vi "单板信息.vi"(11 "VIC_Receive":refnum<vi>) -> ()   [LabVIEW 2013]
panel:
  in  "从板板号 2":u8=1 caption="从板板号" min=1 max=30
  out "滑动杆":dbl(slide)=90.0 caption="SOC" scale=0.0..100.0 scale format="%#_6f"
  out "5":T1
  out "4":T2
  out "3":T3
  out "2":T4
  out "平均电流(A)":dbl
  out "外总压(V)":dbl
  out "总电流(A)":dbl
  out "协议是否公开":string="是"
  out "波特率":string="500Kbps"
  out "应用类型":string
  out "协议版本号":string
  out "SOH":dbl(slide)=30.0 scale=0.0..100.0 scale format="%#_6f"
  in  "刷新":bool
  in  "布尔 3":bool
  out "故障信息":string
  out "最小内阻位置":i32
  out "最大内阻位置":i32
  out "最小内阻":dbl
  out "最大内阻":dbl
  out "最低温度位置":i32
  out "最高温度位置":i32
  out "最低温度":dbl
  out "最高温度":dbl
  out "最低电压位置":i32
  out "最高电压位置":i32
  out "最低电压":dbl
  out "最高电压":dbl
  in  "主界面选项":enum32{"单选选项1", "单选选项2", "单选选项2 2"}(radio)
  in  "继电器状态 2":string[][](table)=[["RL1_ST", "", "RL5_ST"], ["RL2_ST", "", "RL6_ST"], ["RL3_ST", "", "RL7_ST"], ["RL4_ST", "", "RL8_ST"]]
  out "快换帧":T5
  out "从板参数":T6={"总电压"=0.0, "总电流"=0.0, "外总压"=0.0, "平均电流"=0.0, "SOC"=60.0, "SOH"=60.0, "最高电压"=0.0, "位置"=0.0, "最低电压"=0.0, "位置"=0.0, "压差"=0.0, "最高温度"=0.0, "位置"=0.0, "最低温度"=0.0, "位置"=0.0, "最大内阻"=0.0, "位置"=0.0, "最小内阻"=0.0, "位置"=0.0, "故障信息"="", "协议版本号"="", "应用类型"="", "波特率"="", "协议是否公开"="", "电池运行状态"="", "电池充满标志位"="", "Life:"=25.0} {"SOH" scale=0.0..100.0 scale format="%#.0f"; "SOC" scale=0.0..100.0 scale format="%#.0f"}
  out "Life:":dbl=25.0
  out "状态":bool
  out "高压板参数":T7={"总电压"=0.0, "总电流"=0.0, "外总压"=0.0, "平均电流"=0.0, "功率"=0.0, "总充电安时"=0.0, "总放电安时"=0.0, "故障信息"="", "协议版本号"="", "应用类型"="", "波特率"="", "协议是否公开"="", "电池运行状态"="", "Life:"=25.0, "正绝缘电阻"=0.0, "负绝缘电阻"=0.0} {"负绝缘电阻" format="%#.0f"; "正绝缘电阻" format="%#.0f"; "总放电安时" format="%#.0f"; "总充电安时" format="%#.0f"}
  out "继电器颜色":u32[](array[colorbox])
  out "继电器状态":string[](array[string])
  in  "选项卡控件":enum32{"从板监控", "从板信息2", "电压温度", "高压板监控"}(tab)=enum."从板信息2"
  out "从板参数":T8={"最高电压"=0.0, "位置1"=0.0, "最低电压"=0.0, "位置2"=0.0, "压差"=0.0, "最高温度"=0.0, "位置3"=0.0, "最低温度"=0.0, "位置4"=0.0, "温差"=0.0, "最高内阻"=0.0, "位置5"=0.0, "最低内阻"=0.0, "位置6"=0.0, "故障信息"="00", "最大充电总电压"=0.0, "最大充电电流"=0.0, "充电总安时"=0.0, "SOH 2"=0.0, "RL1_ST(fan)"="", "RL2_ST(heat)"="", "RL3_ST"="", "RL4_ST"="", "RL5_ST"="", "RL6_ST"="", "RL7_ST"="", "RL8_ST"=""}
  out "电池充满标志位":string="是"
  out "电池运行状态":string="00"
  out "总电压(V)":dbl
  out "硬件故障":string[][](array[string])
  in  "欠压":u16(ring)
  in  "过压":u16(ring)
  in  "无效":u16(ring)
  in  "故障":u16(ring)
  in  "正常":u16(ring)
  out "供电电源电压(V)":string="0"
  out "内网总线负载率":string="0"
  out "供电电源状态":u16(ring)=1
  out "Flash存储器状态":u16(ring)
  out "外部EE存储器状态":u16(ring)=1
  out "内部EE存储器状态":u16(ring)=3
  out "系统时钟状态":u16(ring)
  out "内部总电压检测模块状态":u16(ring)
  out "外部总电压检测模块状态":u16(ring)
  out "绝缘检测模块状态":u16(ring)
  out "电流模块模块状态":u16(ring)=1 caption="电流检测模块状态"
  out "电池充电均衡模块状态":u16(ring)
  out "电池放电均衡模块状态":u16(ring)=1
  out "温度模块检测状态":u16(ring)=3 caption="温度检测模块状态"
  out "电压模块检测状态":u16(ring) caption="电压检测模块状态"
  in  "偏差":dbl=10.0 format="%#.0f"
  in  "温度基准":dbl=25.0 format="%#.0f"
  in  "布尔 2":bool caption="判定"
  in  "偏差":dbl=0.05 format="%.3f"
  in  "电压基准":dbl=3.7 format="%.3f"
  in  "布尔":bool caption="判定"
  out "1":T9 {"第12串" format="%#.2f"; "第11串" format="%#.2f"; "第10串" format="%#.2f"; "第9串" format="%#.2f"; "第8串" format="%#.2f"; "第7串" format="%#.2f"; "第6串" format="%#.2f"; "第5串" format="%#.2f"; "第4串" format="%#.2f"; "第3串" format="%#.2f"; "第2串" format="%#.2f"; "第1串" format="%#.2f"}
  out "1 7":T1 {"第60串" format="%.3f"; "第59串" format="%.3f"; "第58串" format="%.3f"; "第57串" format="%.3f"; "第56串" format="%.3f"; "第55串" format="%.3f"; "第54串" format="%.3f"; "第53串" format="%.3f"; "第52串" format="%.3f"; "第51串" format="%.3f"; "第50串" format="%.3f"; "第49串" format="%.3f"}
  out "1 6":T2 {"第48串" format="%.3f"; "第47串" format="%.3f"; "第46串" format="%.3f"; "第45串" format="%.3f"; "第44串" format="%.3f"; "第43串" format="%.3f"; "第42串" format="%.3f"; "第41串" format="%.3f"; "第40串" format="%.3f"; "第39串" format="%.3f"; "第38串" format="%.3f"; "第37串" format="%.3f"}
  out "1 4":T3 {"第36串" format="%.3f"; "第35串" format="%.3f"; "第34串" format="%.3f"; "第33串" format="%.3f"; "第32串" format="%.3f"; "第31串" format="%.3f"; "第30串" format="%.3f"; "第29串" format="%.3f"; "第28串" format="%.3f"; "第27串" format="%.3f"; "第26串" format="%.3f"; "第25串" format="%.3f"}
  out "1 3":T4 {"第24串" format="%.3f"; "第23串" format="%.3f"; "第22串" format="%.3f"; "第21串" format="%.3f"; "第20串" format="%.3f"; "第19串" format="%.3f"; "第18串" format="%.3f"; "第17串" format="%.3f"; "第16串" format="%.3f"; "第15串" format="%.3f"; "第14串" format="%.3f"; "第13串" format="%.3f"}
  out "1 102":T9 {"第12串" format="%.3f"; "第11串" format="%.3f"; "第10串" format="%.3f"; "第9串" format="%.3f"; "第8串" format="%.3f"; "第7串" format="%.3f"; "第6串" format="%.3f"; "第5串" format="%.3f"; "第4串" format="%.3f"; "第3串" format="%.3f"; "第2串" format="%.3f"; "第1串" format="%.3f"}
  out "高压板监控":T10={"总电压"=0.0, "总电流"=0.0, "外总压"=0.0, "平均电流"=0.0, "功率"=0.0, "总充电安时"=0.0, "总放电安时"=0.0, "正绝缘电阻"=0.0, "负绝缘电阻"=0.0, "版本协议号"="V1.2.34", "应用类型"="纯电动", "波特率"="500Kbps", "协议是否公开"="是", "故障信息"="00", "电池运行情况"="00"}
  in  "VCI_Receive":T11 {"Rsv3" max=0 format="%x"; "Rsv2" min=101 format="%x"; "Rsv1" format="%x"; "Data8" format="%x"; "Data7" format="%x"; "Data6" format="%x"; "Data5" format="%x"; "Data4" format="%x"; "Data3" format="%x"; "Data2" format="%x"; "Data1" format="%x"; "DataLen" format="%x"; "ExternFlag" format="%x"; "RemoteFlag" format="%x"; "SendType" format="%x"; "TimeFlag" format="%x"; "TimeStamp" format="%x"; "ID" format="%x"}
  in  "停止":bool
  out "单选选项2":bool
  # "从板继电器"
  # "Change frame"
  # "图例"
  # "CellV"
  # "Temp"
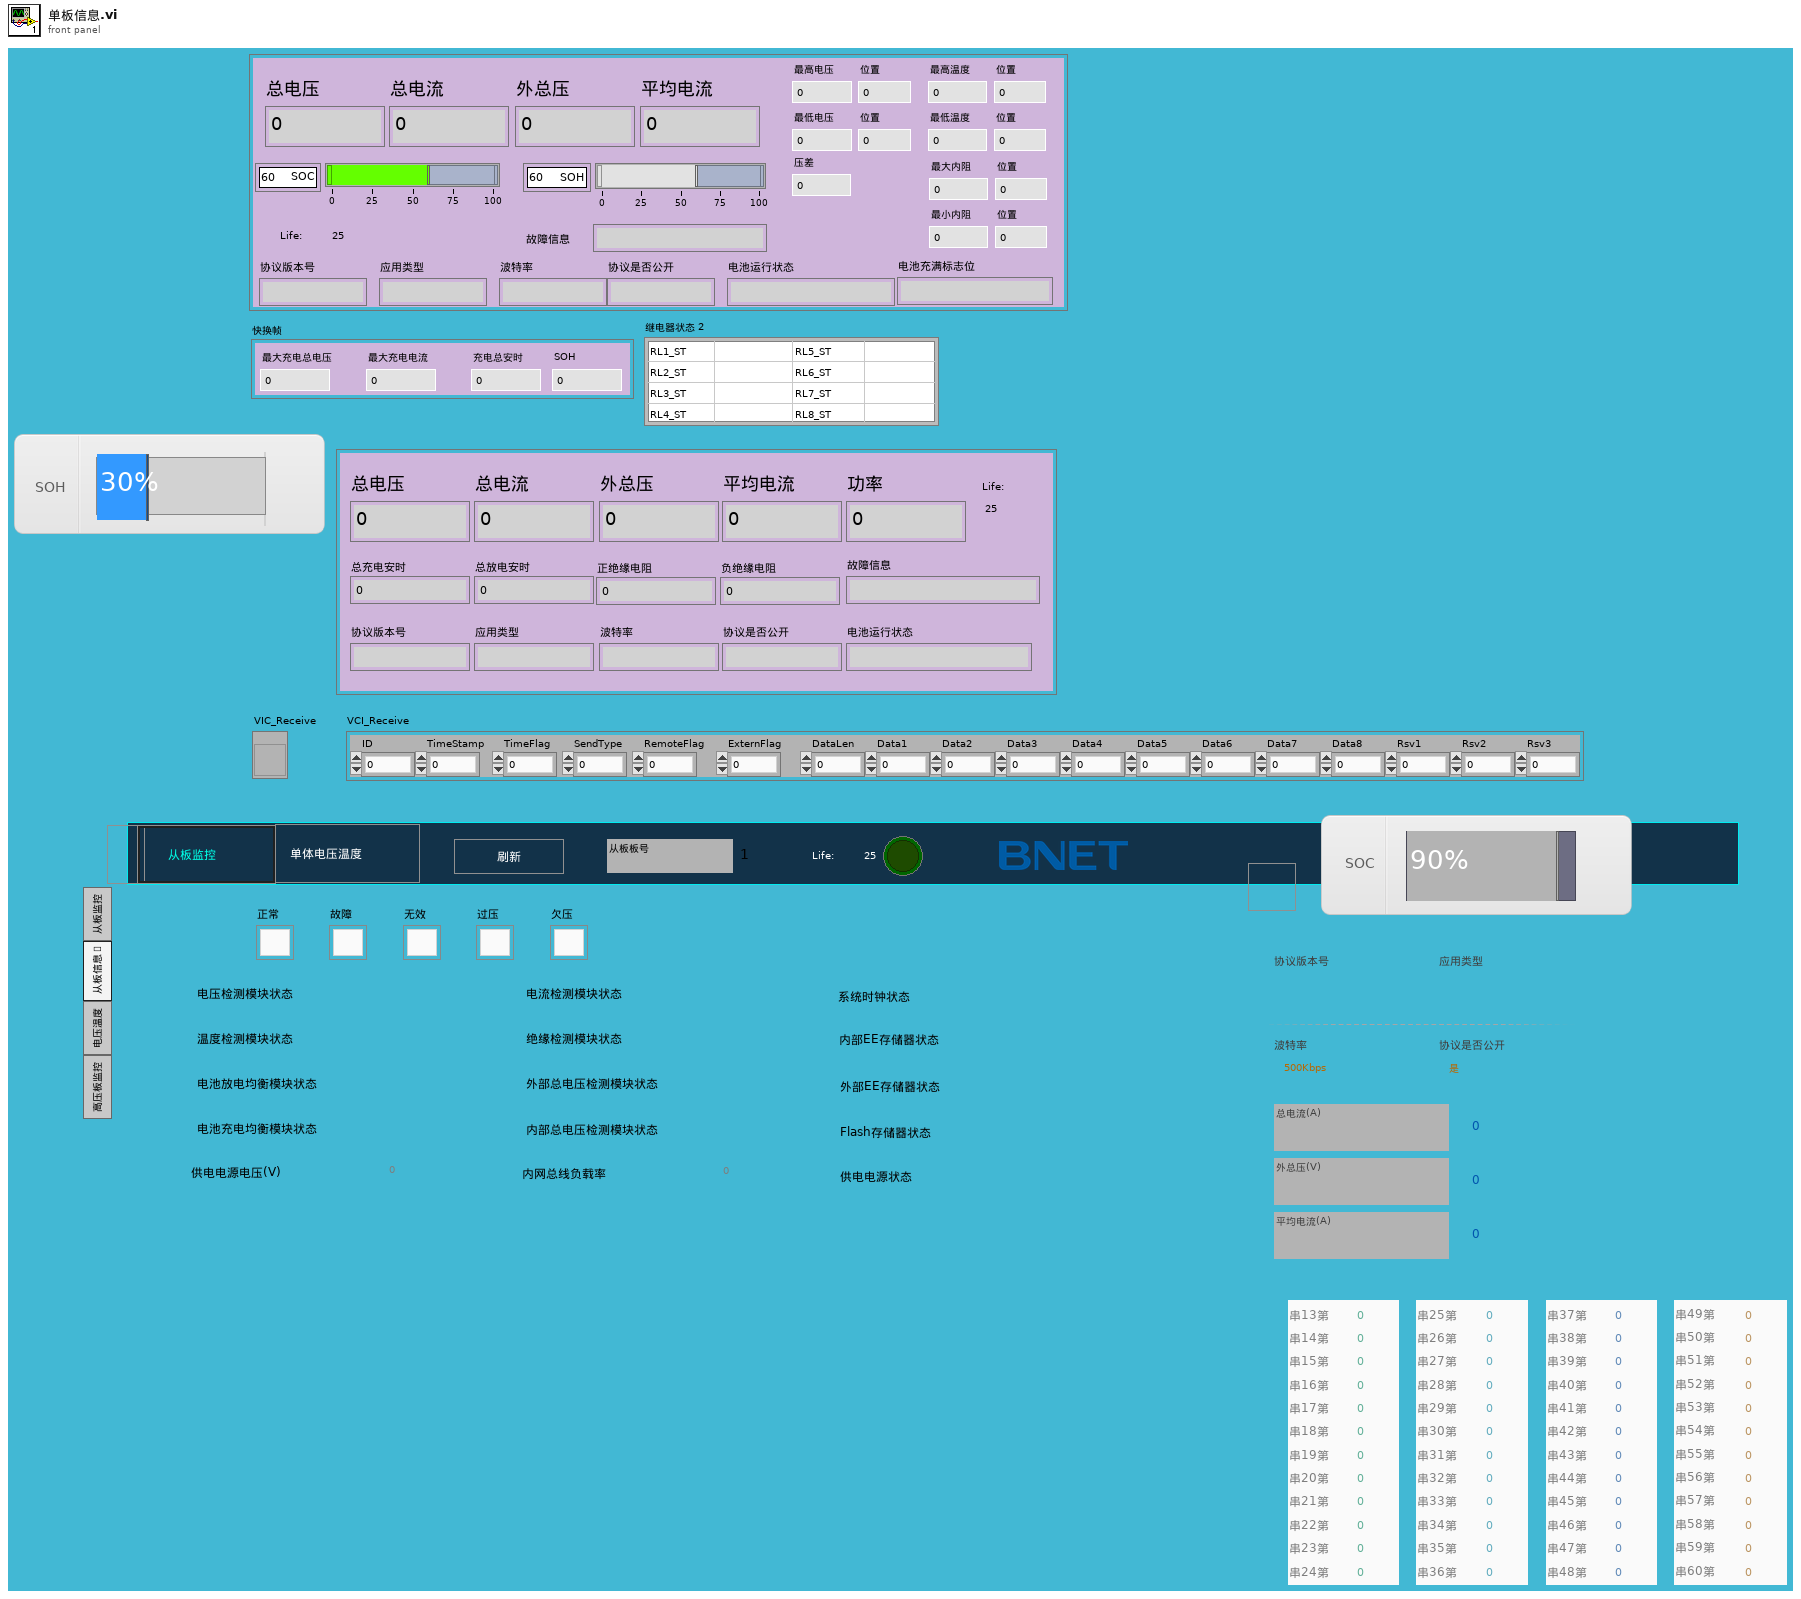
[diagram p1: front panel]
types:
  T1 = cluster{"第49串":dbl, "第50串":dbl, "第51串":dbl, "第52串":dbl, "第53串":dbl, "第54串":dbl, "第55串":dbl, "第56串":dbl, "第57串":dbl, "第58串":dbl, "第59串":dbl, "第60串":dbl}
  T2 = cluster{"第37串":dbl, "第38串":dbl, "第39串":dbl, "第40串":dbl, "第41串":dbl, "第42串":dbl, "第43串":dbl, "第44串":dbl, "第45串":dbl, "第46串":dbl, "第47串":dbl, "第48串":dbl}
  T3 = cluster{"第25串":dbl, "第26串":dbl, "第27串":dbl, "第28串":dbl, "第29串":dbl, "第30串":dbl, "第31串":dbl, "第32串":dbl, "第33串":dbl, "第34串":dbl, "第35串":dbl, "第36串":dbl}
  T4 = cluster{"第13串":dbl, "第14串":dbl, "第15串":dbl, "第16串":dbl, "第17串":dbl, "第18串":dbl, "第19串":dbl, "第20串":dbl, "第21串":dbl, "第22串":dbl, "第23串":dbl, "第24串":dbl}
  T5 = cluster{"SOH":dbl, "充电总安时":dbl, "最大充电电流":dbl, "最大充电总电压":dbl}
  T6 = cluster{"总电压":dbl, "总电流":dbl, "外总压":dbl, "平均电流":dbl, "SOC":dbl, "SOH":dbl, "最高电压":dbl, "位置":dbl, "最低电压":dbl, "位置":dbl, "压差":dbl, "最高温度":dbl, "位置":dbl, "最低温度":dbl, "位置":dbl, "最大内阻":dbl, "位置":dbl, "最小内阻":dbl, "位置":dbl, "故障信息":string, "协议版本号":string, "应用类型":string, "波特率":string, "协议是否公开":string, "电池运行状态":string, "电池充满标志位":string, "Life:":dbl}
  T7 = cluster{"总电压":dbl, "总电流":dbl, "外总压":dbl, "平均电流":dbl, "功率":dbl, "总充电安时":dbl, "总放电安时":dbl, "故障信息":string, "协议版本号":string, "应用类型":string, "波特率":string, "协议是否公开":string, "电池运行状态":string, "Life:":dbl, "正绝缘电阻":dbl, "负绝缘电阻":dbl}
  T8 = cluster{"最高电压":dbl, "位置1":dbl, "最低电压":dbl, "位置2":dbl, "压差":dbl, "最高温度":dbl, "位置3":dbl, "最低温度":dbl, "位置4":dbl, "温差":dbl, "最高内阻":dbl, "位置5":dbl, "最低内阻":dbl, "位置6":dbl, "故障信息":string, "最大充电总电压":dbl, "最大充电电流":dbl, "充电总安时":dbl, "SOH 2":dbl, "RL1_ST(fan)":string, "RL2_ST(heat)":string, "RL3_ST":string, "RL4_ST":string, "RL5_ST":string, "RL6_ST":string, "RL7_ST":string, "RL8_ST":string}
  T9 = cluster{"第1串":dbl, "第2串":dbl, "第3串":dbl, "第4串":dbl, "第5串":dbl, "第6串":dbl, "第7串":dbl, "第8串":dbl, "第9串":dbl, "第10串":dbl, "第11串":dbl, "第12串":dbl}
  T10 = cluster{"总电压":dbl, "总电流":dbl, "外总压":dbl, "平均电流":dbl, "功率":dbl, "总充电安时":dbl, "总放电安时":dbl, "正绝缘电阻":dbl, "负绝缘电阻":dbl, "版本协议号":string, "应用类型":string, "波特率":string, "协议是否公开":string, "故障信息":string, "电池运行情况":string}
  T11 = cluster{"ID":u32, "TimeStamp":u32, "TimeFlag":u8, "SendType":u8, "RemoteFlag":u8, "ExternFlag":u8, "DataLen":u8, "Data1":u8, "Data2":u8, "Data3":u8, "Data4":u8, "Data5":u8, "Data6":u8, "Data7":u8, "Data8":u8, "Rsv1":u8, "Rsv2":u8, "Rsv3":u8}
  T12 = cluster{dbl, dbl, dbl, dbl, dbl, dbl, dbl, dbl, dbl, dbl, dbl, dbl, dbl, dbl, "故障信息":string, dbl, dbl, dbl, dbl, "RL1_ST":string, "RL2_ST":string, "RL3_ST":string, "RL4_ST":string, "RL5_ST":string, "RL6_ST":string, "RL7_ST":string, "RL8_ST":string}
  T13 = enum32{"Invalid", "Standard", "Closed", "Hidden", "Minimized", "Maximized"}
  T14 = cluster{"[0]":dbl, "[1]":dbl, "[2]":dbl, "[3]":dbl, "[4]":dbl, "[5]":dbl, "[6]":dbl, "[7]":dbl, "[8]":dbl, "[9]":dbl, "[10]":dbl, "[11]":dbl}
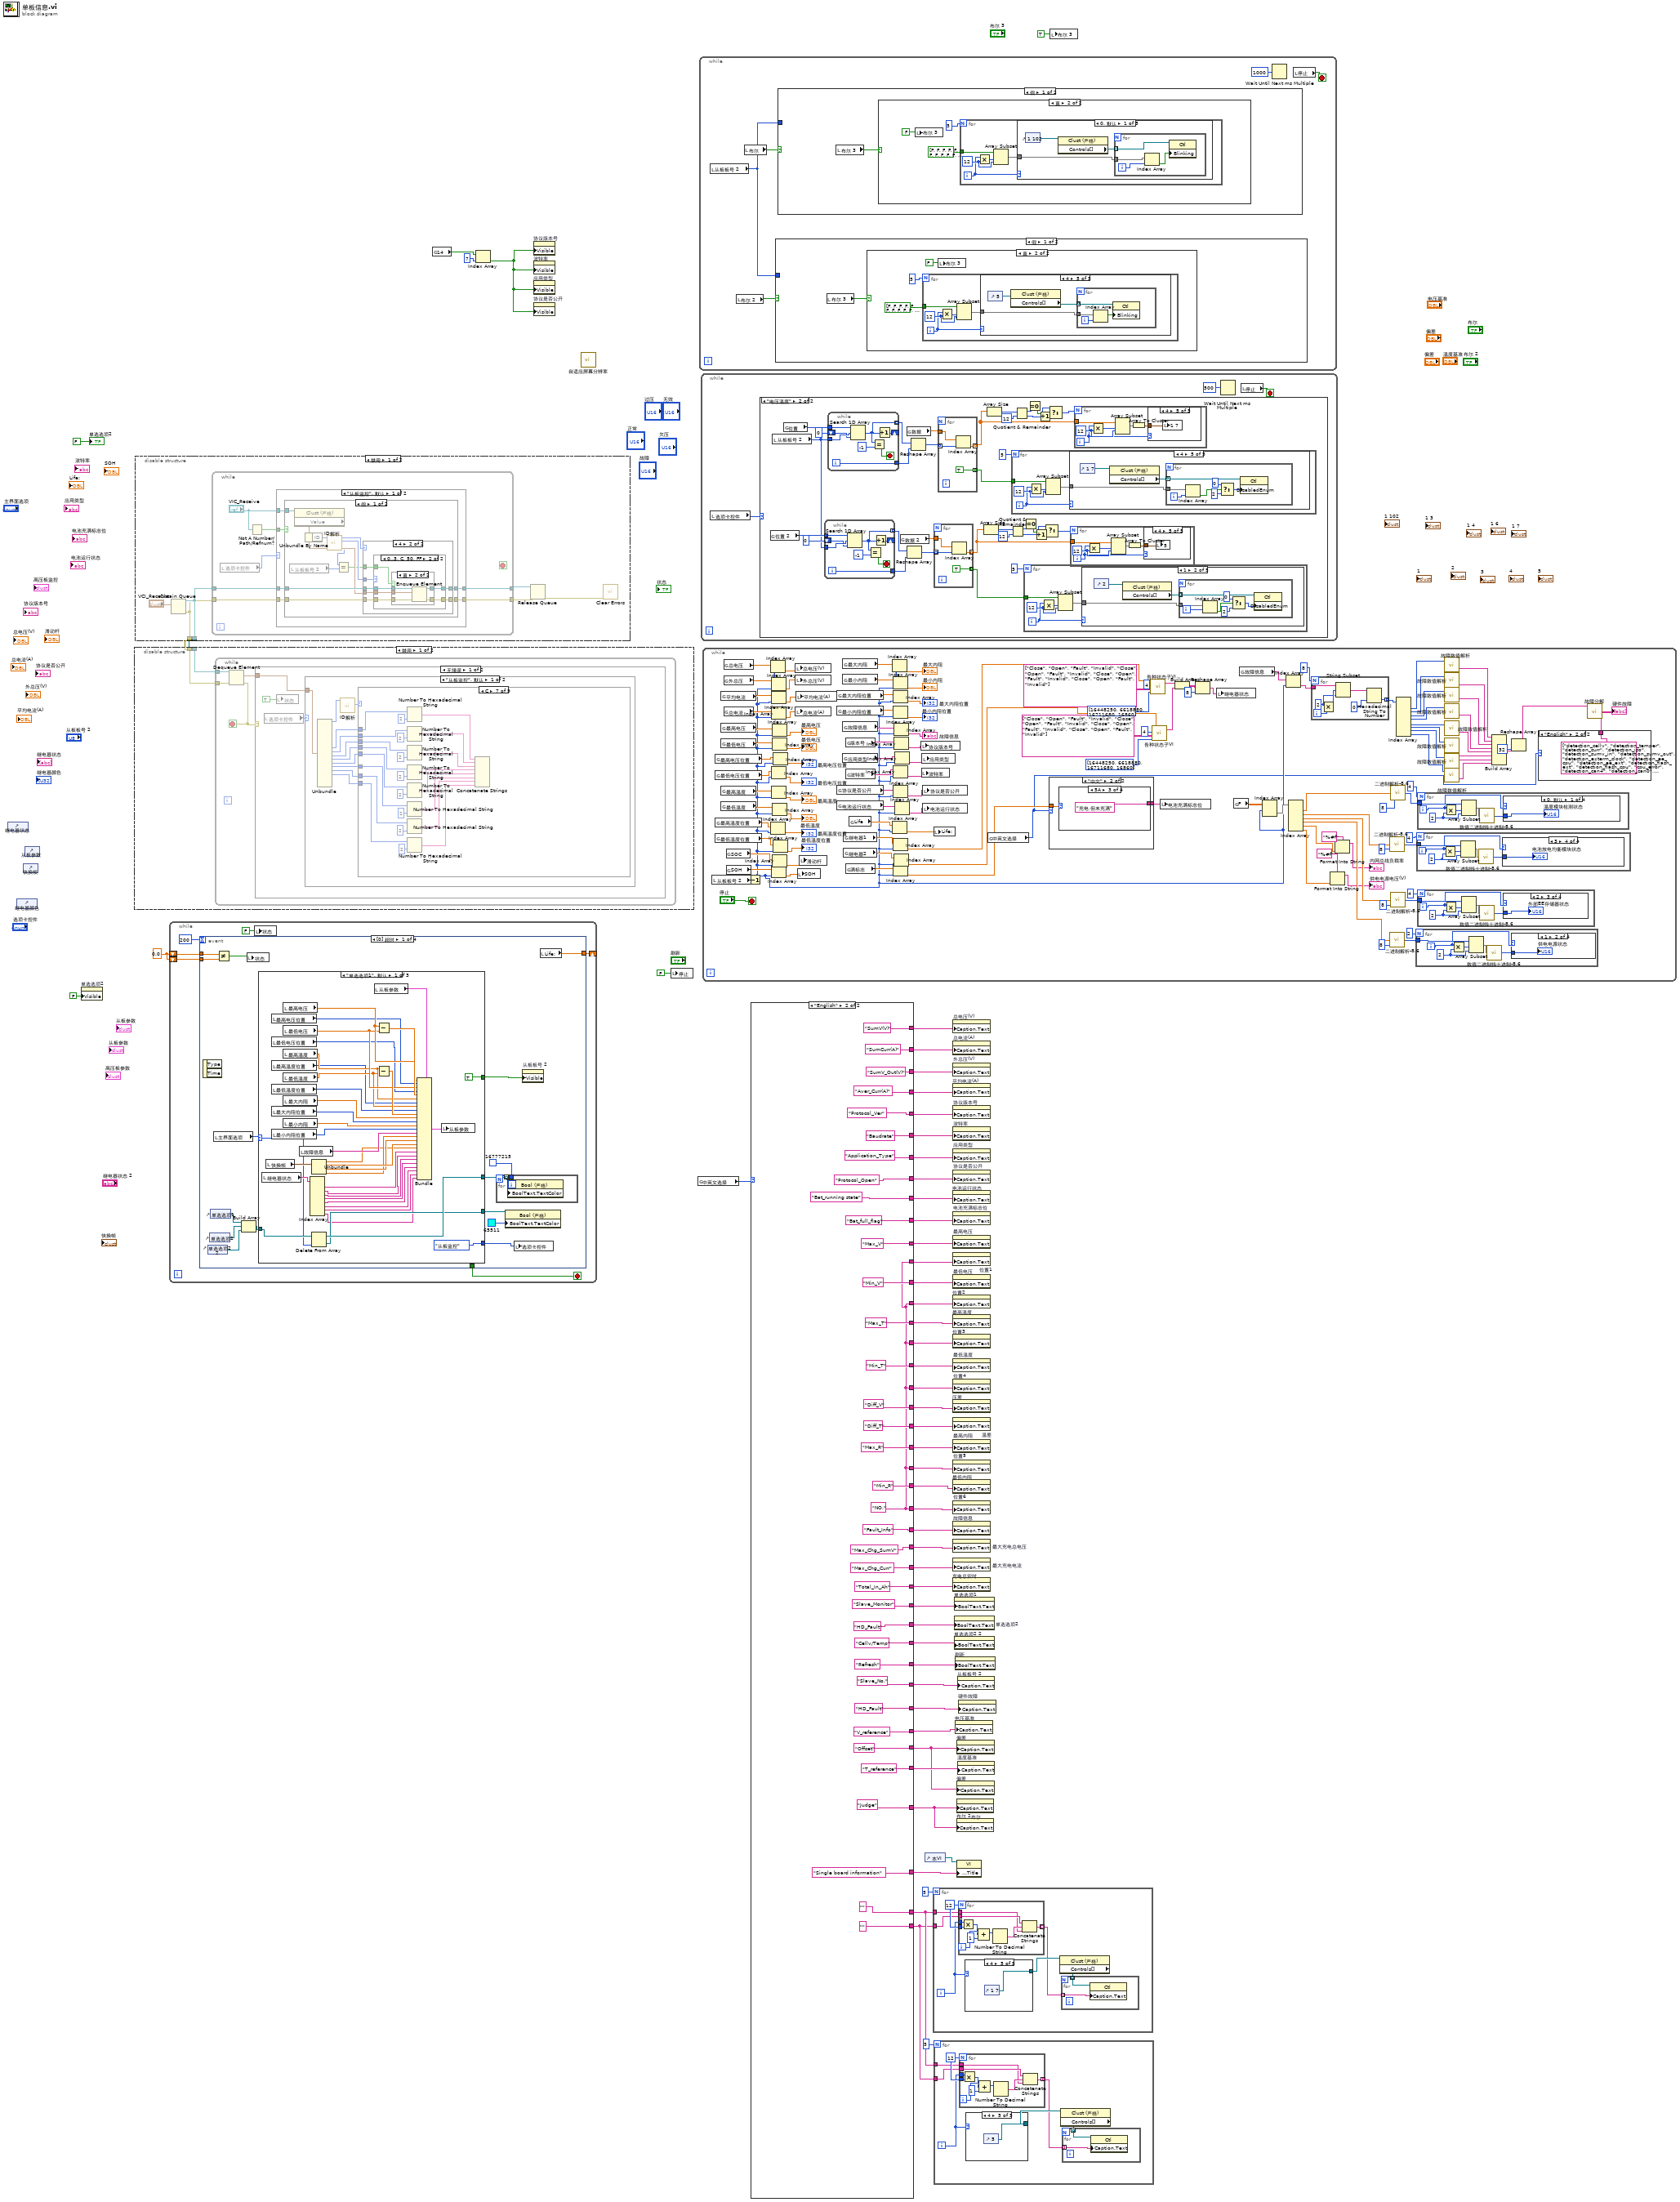
[diagram p0: block diagram]
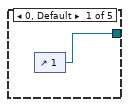
[diagram p2: hidden frame]
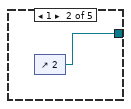
[diagram p3: hidden frame]
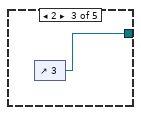
[diagram p4: hidden frame]
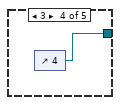
[diagram p5: hidden frame]
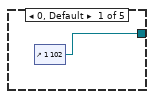
[diagram p6: hidden frame]
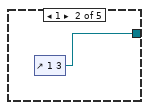
[diagram p7: hidden frame]
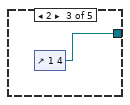
[diagram p8: hidden frame]
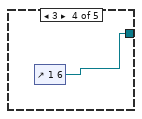
[diagram p9: hidden frame]
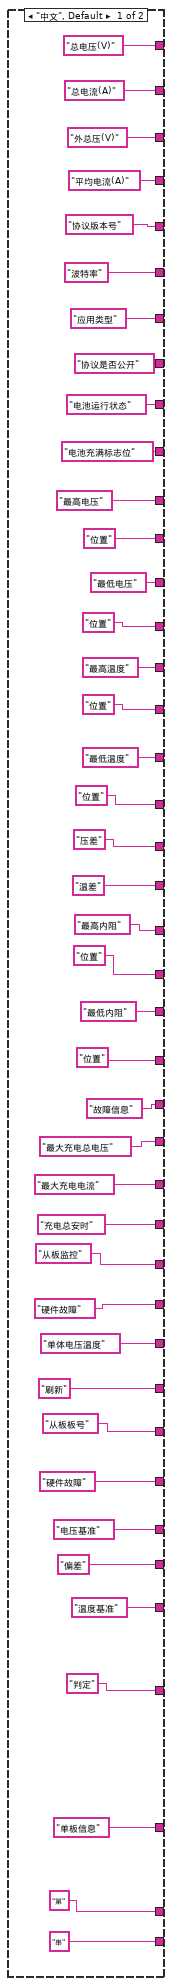
[diagram p10: hidden frame]
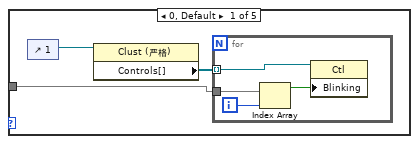
[diagram p12: hidden frame]
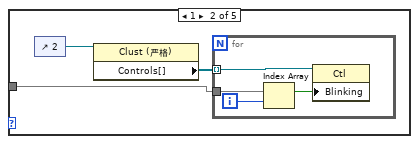
[diagram p13: hidden frame]
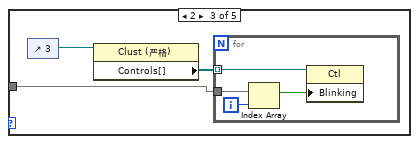
[diagram p14: hidden frame]
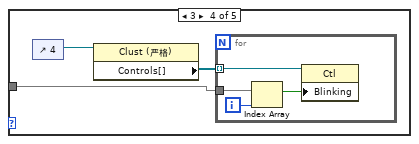
[diagram p15: hidden frame]
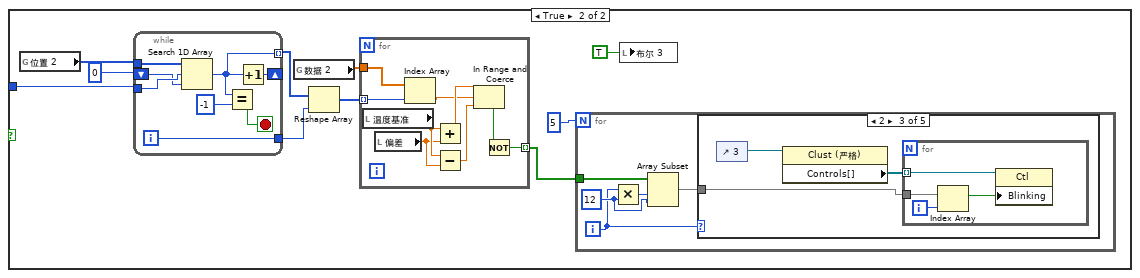
[diagram p16: hidden frame]
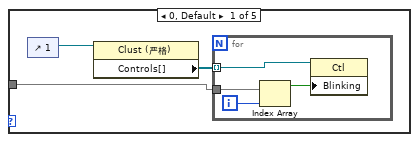
[diagram p17: hidden frame]
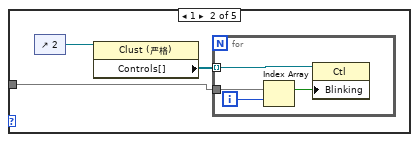
[diagram p18: hidden frame]
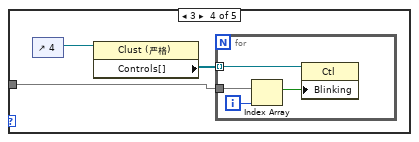
[diagram p19: hidden frame]
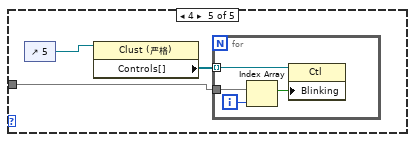
[diagram p20: hidden frame]
diagram:
  w50 = 0.0 ("Life:")
  n1 = control-ref of="继电器状态"() -> ()  [unwired: 1 out]
  n2 = control-ref of="继电器颜色"() -> ()  [unwired: 1 out]
  n3 = control-ref of="快换帧"() -> ()  [unwired: 1 out]
  n4 = control-ref of="从板参数"() -> ()  [unwired: 1 out]
  n5 = property on="单选选项2" class="Bool (严格)"("Visible"=FALSE ("可见")) -> ()  [unwired: 2 in, 2 out]
  n6 = disable-structure shown="禁用" {
    disable-tunnel: [w60 _] -> w55
    disable-tunnel: [w59 _] -> w54
    frame Disabled {
      n7 = Obtain Queue(element data type="VCI_Receive") -> (queue out=w60:refnum<queue>, error out=w59:errorcluster)  [unwired: 4 in, 1 out]
      n8 = while {
        tunnel: w60 -> [w67]
        tunnel: w59 -> [w66]
        tunnel: [w65] -> w58
        tunnel: [w64] -> w57
        stop <- w68 stop-if-true
        n9 = local read "选项卡控件"() -> (w62:enum32{"从板监控", "从板信息2", "电压温度", "高压板监控"})
        n10 = Not A Number/Path/Refnum?(number/path/refnum="VIC_Receive") -> (NaN/Path/Refnum?=w63:bool)
        n11 = case shown="\"从板监控\", 默认" w62 {
          tunnel: "VIC_Receive" -> [w75 w120]
          tunnel: w67 -> [w74 w119]
          tunnel: w66 -> [w73 w118]
          tunnel: [w72 w117] -> w65
          tunnel: [w71 w116] -> w64
          tunnel: w63 -> [w70 w115]
          frame "从板监控", Default {
            n12 = case shown="假" w70 {
              tunnel: w74 -> [w86 w114]
              tunnel: w73 -> [w85 w113]
              tunnel: [w83 w114] -> w72
              tunnel: [w82 w113] -> w71
              tunnel: w75 -> [w81 _]
              frame False {
                n13 = local read "从板板号 2"() -> (w76:u8)
                n14 = property class="Clust (严格)"(reference=w81) -> ("Value"=w84:T11)  [unwired: 1 in, 2 out]
                n15 = Unbundle By Name(w84) -> ("ID"=w87:u32)
                n16 = call "ID解析.vi"("ID"=w87) -> ("SA(4)"=w78:i32, "PF(2)"=w79:i32, "PDU(1)"=w80:i32)  [unwired: 8 out]
                n17 = Equal?(x=w78, y=w76) -> (x = y?=w77:bool)
                n18 = case shown="4" w80 {
                  tunnel: w86 -> [w89 w96]
                  tunnel: w85 -> [w88 w95]
                  tunnel: w84 -> [_ w94]
                  tunnel: [w89 w93] -> w83
                  tunnel: [w88 w92] -> w82
                  tunnel: w79 -> [_ w91]
                  tunnel: w77 -> [_ w90]
                  frame 0, Default {
                  }
                  frame 4 {
                    n19 = case shown="0..3, C, 50, FF" w91 {
                      tunnel: w96 -> [w98 w104]
                      tunnel: w95 -> [w97 w103]
                      tunnel: w94 -> [_ w102]
                      tunnel: [w98 w101] -> w93
                      tunnel: [w97 w100] -> w92
                      tunnel: w90 -> [_ w99]
                      frame 153, Default {
                      }
                      frame 0..3, 12, 80, 255 {
                        n20 = case shown="真" w99 {
                          tunnel: w104 -> [w106 w111]
                          tunnel: w103 -> [w105 w110]
                          tunnel: w102 -> [_ w109]
                          tunnel: [w106 w108] -> w101
                          tunnel: [w105 w107] -> w100
                          frame False {
                          }
                          frame True {
                            n21 = Enqueue Element(queue=w111, element=w109, error in (no error)=w110) -> (queue out=w108:refnum<queue>, error out=w107:errorcluster)  [unwired: 2 out]
                          }
                        }
                      }
                    }
                  }
                }
              }
              frame True {
                n22 = Wait Until Next ms Multiple(millisecond multiple=u32 100 ("毫秒倍数")) -> ()  [unwired: 1 out]
              }
            }
          }
          frame "高压板监控" {
            n23 = case shown="假" w115 {
              tunnel: w119 -> [w132 w160]
              tunnel: w118 -> [w131 w159]
              tunnel: [w129 w160] -> w117
              tunnel: [w128 w159] -> w116
              tunnel: w120 -> [w127 _]
              frame False {
                n24 = property class="Clust (严格)"(reference=w127) -> ("Value"=w130:T11)  [unwired: 1 in, 2 out]
                n25 = Unbundle By Name(w130) -> ("ID"=w133:u32)
                n26 = call "ID解析.vi"("ID"=w133) -> ("SA(4)"=w124:i32, "PF(2)"=w125:i32, "PDU(1)"=w126:i32)  [unwired: 8 out]
                n27 = Equal?(x=w124, y=62) -> (x = y?=w123:bool)
                n28 = case shown="4" w126 {
                  tunnel: w132 -> [w135 w142]
                  tunnel: w131 -> [w134 w141]
                  tunnel: w130 -> [_ w140]
                  tunnel: [w135 w139] -> w129
                  tunnel: [w134 w138] -> w128
                  tunnel: w125 -> [_ w137]
                  tunnel: w123 -> [_ w136]
                  frame 0, Default {
                  }
                  frame 4 {
                    n29 = case shown="0, 5, 8, C, FF" w137 {
                      tunnel: w142 -> [w144 w150]
                      tunnel: w141 -> [w143 w149]
                      tunnel: w140 -> [_ w148]
                      tunnel: [w144 w147] -> w139
                      tunnel: [w143 w146] -> w138
                      tunnel: w136 -> [_ w145]
                      frame 153, Default {
                      }
                      frame 0, 5, 8, 12, 255 {
                        n30 = case shown="真" w145 {
                          tunnel: w150 -> [w152 w157]
                          tunnel: w149 -> [w151 w156]
                          tunnel: w148 -> [_ w155]
                          tunnel: [w152 w154] -> w147
                          tunnel: [w151 w153] -> w146
                          frame False {
                          }
                          frame True {
                            n31 = Enqueue Element(queue=w157, element=w155, error in (no error)=w156) -> (queue out=w154:refnum<queue>, error out=w153:errorcluster)  [unwired: 2 out]
                          }
                        }
                      }
                    }
                  }
                }
                n32 = local write "状态"(FALSE ("接收")) -> ()
              }
              frame True {
                n33 = Wait Until Next ms Multiple(millisecond multiple=u32 100 ("毫秒倍数")) -> ()  [unwired: 1 out]
              }
            }
          }
        }
      }
      n34 = Release Queue(queue=w58, error in (no error)=w57) -> (error out=w56:errorcluster)  [unwired: 3 out]
      n35 = call <vilib>:"Clear Errors.vi"("error in (no error)"=w56) -> ()  [unwired: 7 out]
    }
    frame Enabled {
    }
  }
  n36 = disable-structure shown="禁用" {
    disable-tunnel: w55 -> [w162 _]
    disable-tunnel: w54 -> [w161 _]
    frame Disabled {
      n37 = while {
        tunnel: w162 -> [w165]
        tunnel: w161 -> [w164]
        stop <- w166 stop-if-true
        n38 = Dequeue Element(queue=w165, error in (no error)=w164) -> (element=w163:T11, error out=w166:errorcluster)  [unwired: 3 out]
        n39 = case shown="无错误" w166 {
          tunnel: w163 -> [w169 _]
          frame No Error {
            n40 = local read "选项卡控件"() -> (w168:enum32{"从板监控", "从板信息2", "电压温度", "高压板监控"})
            n41 = local write "状态"(TRUE ("接收")) -> ()
            n42 = case shown="\"从板监控\", 默认" w168 {
              tunnel: w169 -> [w180 w366]
              frame "从板监控", Default {
                n43 = Unbundle(w180) -> ("ID"=w179:u32, "Data1"=w177:u8, "Data2"=w176:u8, "Data3"=w175:u8, "Data4"=w174:u8, "Data5"=w173:u8, "Data6"=w172:u8, "Data7"=w171:u8, "Data8"=w170:u8)  [unwired: 9 out]
                n44 = call "ID解析.vi"("ID"=w179) -> ("PF(2)"=w178:i32)  [unwired: 10 out]
                n45 = case shown="C" w178 {
                  tunnel: w177 -> [_ w190 w219 w233 w255 w287 w307 w325 w330]
                  tunnel: w176 -> [_ w189 w218 w232 w254 w286 w306 _ w329]
                  tunnel: w175 -> [_ w188 w217 w231 w253 w285 w305 _ w328]
                  tunnel: w174 -> [_ w187 w216 w230 w252 w284 w304 _ _]
                  tunnel: w173 -> [_ w186 w215 w229 w251 w283 w303 _ w327]
                  tunnel: w172 -> [_ w185 w214 w228 w250 w282 w302 w324 _]
                  tunnel: w171 -> [_ w184 w201 w227 w249 w281 w301 _ _]
                  tunnel: w170 -> [_ w183 w200 _ w248 _ w300 _ w326]
                  frame 153, Default {
                    n46 = Wait Until Next ms Multiple(millisecond multiple=u32 2 ("毫秒倍数")) -> ()  [unwired: 1 out]
                  }
                  frame 0 {
                    n47 = Join Numbers(hi=w188, lo=w187) -> ((hi.lo)=w195:u16)
                    n48 = Join Numbers(hi=w186, lo=w185) -> ((hi.lo)=w197:u16)
                    n49 = Join Numbers(hi=w190, lo=w189) -> ((hi.lo)=w196:u16)
                    n50 = Join Numbers(hi=w184, lo=w183) -> ((hi.lo)=w191:u16)
                    n51 = call "输出分辨率计算.vi"("偏移量"=sgl -3000.0, "分辨率"=0.1, "数值 3"=w195, "数值 2"=w191) -> ()  [unwired: 2 in, 6 out]
                    n52 = call "输出分辨率计算.vi"("分辨率"=0.1, "数值 3"=w197, "数值 2"=w196) -> ("输出2"=w182:dbl)  [unwired: 3 in, 5 out]
                  }
                  frame 144 {
                    n53 = Join Numbers(hi=w217, lo=w216) -> ((hi.lo)=w223:u16)
                    n54 = Join Numbers(hi=w215, lo=w214) -> ((hi.lo)=w213:u16)
                    n55 = Join Numbers(hi=w219, lo=w218) -> ((hi.lo)=w224:u16)
                    n56 = call "二进制解析-8.6.vi"("索引"=8, "数值"=w201) -> ("低位子数组"=w204:i32[])  [unwired: 3 out]
                    n57 = call "二进制解析-8.6.vi"("索引"=4, "数值"=w200) -> ("高位子数组"=w203:i32[])  [unwired: 3 out]
                    n58 = Insert Into Array(array=w204, new element=w203) -> (w202:i32[])  [unwired: 1 in]
                    n59 = call "输出分辨率计算.vi"("分辨率"=0.001, "数值 2"=w213) -> ("输出2"=w207:dbl)  [unwired: 4 in, 5 out]
                    n60 = local read "快换帧"() -> (w211:T5)
                    n61 = call "数值二进制转十进制-8.6.vi"("子数组"=w202) -> ("十进制数值"=w199:i32)  [unwired: 4 out]
                    n62 = call "输出分辨率计算.vi"("分辨率"=0.1, "数值 3"=w199, "数值 2"=w224) -> ("输出3"=w198:dbl, "输出2"=w208:dbl)  [unwired: 3 in, 4 out]
                    n63 = call "输出分辨率计算.vi"("偏移量"=sgl -3000.0, "分辨率"=0.1, "数值 3"=w223) -> ("输出3"=w209:dbl)  [unwired: 3 in, 5 out]
                    n64 = Bundle(cluster=w211, "SOH"=w198, "充电总安时"=w207, "最大充电电流"=w209, "最大充电总电压"=w208) -> (w210:T5)
                    n65 = local write "快换帧"(w210) -> ()
                  }
                  frame 1 {
                    n66 = Join Numbers(hi=w233, lo=w232) -> ((hi.lo)=w234:u16)
                    n67 = Join Numbers(hi=w231, lo=w230) -> ((hi.lo)=w235:u16)
                    n68 = call "二进制解析-8.6.vi"("索引"=8, "数值"=w227) -> ("低位子数组"=w243:i32[])  [unwired: 3 out]
                    n69 = call "二进制解析-8.6.vi"("索引"=8, "数值"=w229) -> ("低位子数组"=w240:i32[])  [unwired: 3 out]
                    n70 = call "二进制解析-8.6.vi"("索引"=4, "数值"=w228) -> ("低位子数组"=w242:i32[], "高位子数组"=w241:i32[])  [unwired: 2 out]
                    n71 = Insert Into Array(array=w240, new element=w241) -> (w245:i32[])  [unwired: 1 in]
                    n72 = Insert Into Array(array=w242, new element=w243) -> (w244:i32[])  [unwired: 1 in]
                    n73 = call "输出分辨率计算.vi"("分辨率"=0.001, "数值 3"=w235, "数值 2"=w234) -> ("输出3"=w226:dbl, "输出2"=w225:dbl)  [unwired: 3 in, 4 out]
                    n74 = call "数值二进制转十进制-8.6.vi"("子数组"=w245) -> ()  [unwired: 5 out]
                    n75 = call "数值二进制转十进制-8.6.vi"("子数组"=w244) -> ()  [unwired: 5 out]
                  }
                  frame 2 {
                    n76 = call "二进制解析-8.6.vi"("索引"=8, "数值"=w248) -> ("低位子数组"=w269:i32[])  [unwired: 3 out]
                    n77 = call "二进制解析-8.6.vi"("索引"=8, "数值"=w250) -> ("低位子数组"=w272:i32[])  [unwired: 3 out]
                    n78 = call "二进制解析-8.6.vi"("索引"=4, "数值"=w249) -> ("低位子数组"=w270:i32[], "高位子数组"=w271:i32[])  [unwired: 2 out]
                    n79 = call "二进制解析-8.6.vi"("索引"=8, "数值"=w251) -> ("低位子数组"=w263:i32[])  [unwired: 3 out]
                    n80 = call "二进制解析-8.6.vi"("索引"=8, "数值"=w253) -> ("低位子数组"=w260:i32[])  [unwired: 3 out]
                    n81 = call "二进制解析-8.6.vi"("索引"=4, "数值"=w252) -> ("低位子数组"=w262:i32[], "高位子数组"=w261:i32[])  [unwired: 2 out]
                    n82 = call "输出分辨率计算.vi"("偏移量"=sgl -40.0, "分辨率"=1.0, "数值 3"=w254, "数值 2"=w255) -> ()  [unwired: 2 in, 6 out]
                    n83 = Insert Into Array(array=w272, new element=w271) -> (w267:i32[])  [unwired: 1 in]
                    n84 = Insert Into Array(array=w270, new element=w269) -> (w268:i32[])  [unwired: 1 in]
                    n85 = Insert Into Array(array=w260, new element=w261) -> (w265:i32[])  [unwired: 1 in]
                    n86 = Insert Into Array(array=w262, new element=w263) -> (w264:i32[])  [unwired: 1 in]
                    n87 = call "数值二进制转十进制-8.6.vi"("子数组"=w267) -> ("十进制数值"=w276:i32)  [unwired: 4 out]
                    n88 = call "数值二进制转十进制-8.6.vi"("子数组"=w265) -> ()  [unwired: 5 out]
                    n89 = call "数值二进制转十进制-8.6.vi"("子数组"=w268) -> ("十进制数值"=w277:i32)  [unwired: 4 out]
                    n90 = call "数值二进制转十进制-8.6.vi"("子数组"=w264) -> ()  [unwired: 5 out]
                    n91 = call "输出分辨率计算.vi"("分辨率"=0.1, "数值 3"=w277, "数值 2"=w276) -> ("输出3"=w246:dbl, "输出2"=w247:dbl)  [unwired: 3 in, 4 out]
                  }
                  frame 3 {
                    n92 = Join Numbers(hi=w287, lo=w286) -> ((hi.lo)=w288:u16)
                    n93 = Join Numbers(hi=w285, lo=w284) -> ((hi.lo)=w289:u16)
                    n94 = call "二进制解析-8.6.vi"("索引"=8, "数值"=w281) -> ("低位子数组"=w297:i32[])  [unwired: 3 out]
                    n95 = call "二进制解析-8.6.vi"("索引"=8, "数值"=w283) -> ("低位子数组"=w294:i32[])  [unwired: 3 out]
                    n96 = call "二进制解析-8.6.vi"("索引"=4, "数值"=w282) -> ("低位子数组"=w296:i32[], "高位子数组"=w295:i32[])  [unwired: 2 out]
                    n97 = Insert Into Array(array=w294, new element=w295) -> (w299:i32[])  [unwired: 1 in]
                    n98 = Insert Into Array(array=w296, new element=w297) -> (w298:i32[])  [unwired: 1 in]
                    n99 = call "输出分辨率计算.vi"("分辨率"=0.001, "数值 3"=w289, "数值 2"=w288) -> ("输出3"=w279:dbl, "输出2"=w280:dbl)  [unwired: 3 in, 4 out]
                    n100 = call "数值二进制转十进制-8.6.vi"("子数组"=w299) -> ()  [unwired: 5 out]
                    n101 = call "数值二进制转十进制-8.6.vi"("子数组"=w298) -> ()  [unwired: 5 out]
                  }
                  frame 12 {
                    n102 = Number To Hexadecimal String(1:i16 2 ("宽度(-)"), 2:w307) -> (0:w316:string)
                    n103 = Number To Hexadecimal String(1:i16 2 ("宽度(-)"), 2:w306) -> (0:w317:string)
                    n104 = Number To Hexadecimal String(1:i16 2 ("宽度(-)"), 2:w305) -> (0:w318:string)
                    n105 = Number To Hexadecimal String(1:i16 2 ("宽度(-)"), 2:w304) -> (0:w319:string)
                    n106 = Number To Hexadecimal String(1:i16 2 ("宽度(-)"), 2:w303) -> (0:w320:string)
                    n107 = Number To Hexadecimal String(1:i16 2 ("宽度(-)"), 2:w302) -> (0:w321:string)
                    n108 = Number To Hexadecimal String(1:i16 2 ("宽度(-)"), 2:w301) -> (0:w322:string)
                    n109 = Number To Hexadecimal String(1:i16 2 ("宽度(-)"), 2:w300) -> (0:w323:string)
                    n110 = Concatenate Strings(w316, w317, w318, w319, w320, w321, w322, w323) -> ()  [unwired: 1 out]
                  }
                  frame 80 {
                  }
                  frame 255 {
                    n111 = call "二进制解析-8.6.vi"("索引"=4, "数值"=w330) -> ("低位子数组"=w331:i32[], "高位子数组"=w332:i32[])  [unwired: 2 out]
                    n112 = call "二进制解析-8.6.vi"("索引"=6, "数值"=w329) -> ("低位子数组"=w342:i32[], "高位子数组"=w341:i32[])  [unwired: 2 out]
                    n113 = call "二进制解析-8.6.vi"("索引"=7, "数值"=w328) -> ("高位子数组"=w346:i32[])  [unwired: 3 out]
                    n114 = call "数值二进制转十进制-8.6.vi"("子数组"=w342) -> ("十进制数值"=w343:i32)  [unwired: 4 out]
                    n115 = call "数值二进制转十进制-8.6.vi"("子数组"=w331) -> ("十进制数值"=w334:i32)  [unwired: 4 out]
                    n116 = call "数值二进制转十进制-8.6.vi"("子数组"=w341) -> ("十进制数值"=w344:i32)  [unwired: 4 out]
                    n117 = call "数值二进制转十进制-8.6.vi"("子数组"=w346) -> ("十进制数值"=w347:i32)  [unwired: 4 out]
                    n118 = call "数值二进制转十进制-8.6.vi"("子数组"=w332) -> ("十进制数值"=w333:i32)  [unwired: 4 out]
                    n119 = case shown="1" w347 {
                      tunnel: ["不公开" "公开"] -> _
                      frame 0, Default {
                      }
                      frame 1 {
                      }
                    }
                    n120 = case shown="0, 默认" w343 {
                      tunnel: ["500Kps" "250Kps"] -> _
                      frame 0, Default {
                      }
                      frame 1 {
                      }
                    }
                    n121 = Number To Decimal String(number=w333) -> (decimal integer string=w335:string)  [unwired: 1 out]
                    n122 = case shown="4" w344 {
                      tunnel: [_ "纯电动BMS" "混合动力BMS" "储能" "快换"] -> _
                      frame 0, Default {
                      }
                      frame 1 {
                      }
                      frame 2 {
                      }
                      frame 3 {
                      }
                      frame 4 {
                      }
                    }
                    n123 = Number To Decimal String(number=w334) -> (decimal integer string=w337:string)  [unwired: 1 out]
                    n124 = call "运行模式解析.vi"("输入值"=w327) -> ()  [unwired: 1 in, 1 out]
                    n125 = Concatenate Strings("V" ("字符串"), w335, "." ("字符串"), w337) -> ()  [unwired: 1 out]
                  }
                }
              }
              frame "高压板监控" {
                n126 = Unbundle(w366) -> ("ID"=w365:u32, "Data1"=w363:u8, "Data2"=w362:u8, "Data3"=w361:u8, "Data4"=w360:u8, "Data5"=w359:u8, "Data6"=w358:u8, "Data7"=w357:u8, "Data8"=w356:u8)  [unwired: 9 out]
                n127 = call "ID解析.vi"("ID"=w365) -> ("PF(2)"=w364:i32)  [unwired: 10 out]
                n128 = case shown="99, 默认" w364 {
                  tunnel: w363 -> [_ w381 w400 w418 w446]
                  tunnel: w362 -> [_ w380 w399 w417 w445]
                  tunnel: w361 -> [_ w379 w398 w416 w444]
                  tunnel: w360 -> [_ w378 w397 w415 _]
                  tunnel: w359 -> [_ w377 w396 w414 w443]
                  tunnel: w358 -> [_ w376 w395 w413 _]
                  tunnel: w357 -> [_ w375 w394 w412 _]
                  tunnel: w356 -> [_ w374 w393 w411 w442]
                  frame 153, Default {
                    n129 = Wait Until Next ms Multiple(millisecond multiple=u32 2 ("毫秒倍数")) -> ()  [unwired: 1 out]
                  }
                  frame 0 {
                    n130 = Join Numbers(hi=w379, lo=w378) -> ((hi.lo)=w386:u16)
                    n131 = Join Numbers(hi=w377, lo=w376) -> ((hi.lo)=w388:u16)
                    n132 = Join Numbers(hi=w381, lo=w380) -> ((hi.lo)=w387:u16)
                    n133 = Join Numbers(hi=w375, lo=w374) -> ((hi.lo)=w382:u16)
                    n134 = call "输出分辨率计算.vi"("偏移量"=sgl -3000.0, "分辨率"=0.1, "数值 3"=w386, "数值 2"=w382) -> ("输出3"=w368:dbl, "输出2"=w369:dbl)  [unwired: 2 in, 4 out]
                    n135 = call "输出分辨率计算.vi"("分辨率"=0.1, "数值 3"=w388, "数值 2"=w387) -> ("输出3"=w370:dbl, "输出2"=w371:dbl)  [unwired: 3 in, 4 out]
                    n136 = local read "高压板监控"() -> (w373:T10)
                    n137 = Bundle By Name(cluster=w373, "总电压"=w371, "外总压"=w370, "平均电流"=w369, "总电流"=w368) -> (w372:T10)
                    n138 = local write "高压板监控"(w372) -> ()
                  }
                  frame 5 {
                    n139 = Join Numbers(hi=w400, lo=w399) -> ((hi.lo)=w403:u16)
                    n140 = Join Numbers(hi=w398, lo=w397) -> ((hi.lo)=w402:u16)
                    n141 = Join Numbers(hi=w396, lo=w395) -> ((hi.lo)=w404:u16)
                    n142 = Join Numbers(hi=w394, lo=w393) -> ((hi.lo)=w405:u16)
                    n143 = Join Numbers(hi=w403, lo=w402) -> ((hi.lo)=w407:u32)
                    n144 = Join Numbers(hi=w404, lo=w405) -> ((hi.lo)=w406:u32)
                    n145 = call "输出分辨率计算.vi"("分辨率"=0.001, "数值 3"=w406, "数值 2"=w407) -> ("输出3"=w390:dbl, "输出2"=w391:dbl)  [unwired: 3 in, 4 out]
                    n146 = local read "高压板监控"() -> (w392:T10)
                    n147 = Bundle By Name(cluster=w392, "总充电安时"=w391, "总放电安时"=w390) -> (w389:T10)
                    n148 = local write "高压板监控"(w389) -> ()
                  }
                  frame 12 {
                    n149 = Number To Hexadecimal String(1:i16 2 ("宽度(-)"), 2:w418) -> (0:w427:string)
                    n150 = Number To Hexadecimal String(1:i16 2 ("宽度(-)"), 2:w417) -> (0:w428:string)
                    n151 = Number To Hexadecimal String(1:i16 2 ("宽度(-)"), 2:w416) -> (0:w429:string)
                    n152 = Number To Hexadecimal String(1:i16 2 ("宽度(-)"), 2:w415) -> (0:w430:string)
                    n153 = Number To Hexadecimal String(1:i16 2 ("宽度(-)"), 2:w414) -> (0:w431:string)
                    n154 = Number To Hexadecimal String(1:i16 2 ("宽度(-)"), 2:w413) -> (0:w432:string)
                    n155 = Number To Hexadecimal String(1:i16 2 ("宽度(-)"), 2:w412) -> (0:w433:string)
                    n156 = Number To Hexadecimal String(1:i16 2 ("宽度(-)"), 2:w411) -> (0:w434:string)
                    n157 = Concatenate Strings(w427, w428, w429, w430, w431, w432, w433, w434) -> (w409:string)
                    n158 = local read "高压板监控"() -> (w410:T10)
                    n159 = Bundle By Name(cluster=w410, "故障信息"=w409) -> (w408:T10)
                    n160 = local write "高压板监控"(w408) -> ()
                  }
                  frame 255 {
                    n161 = local write "Life:"(w442) -> ()
                    n162 = call "二进制解析-8.6.vi"("索引"=4, "数值"=w446) -> ("低位子数组"=w447:i32[], "高位子数组"=w448:i32[])  [unwired: 2 out]
                    n163 = call "二进制解析-8.6.vi"("索引"=6, "数值"=w445) -> ("低位子数组"=w458:i32[], "高位子数组"=w457:i32[])  [unwired: 2 out]
                    n164 = call "二进制解析-8.6.vi"("索引"=7, "数值"=w444) -> ("高位子数组"=w462:i32[])  [unwired: 3 out]
                    n165 = call "数值二进制转十进制-8.6.vi"("子数组"=w458) -> ("十进制数值"=w459:i32)  [unwired: 4 out]
                    n166 = call "数值二进制转十进制-8.6.vi"("子数组"=w447) -> ("十进制数值"=w450:i32)  [unwired: 4 out]
                    n167 = call "数值二进制转十进制-8.6.vi"("子数组"=w457) -> ("十进制数值"=w460:i32)  [unwired: 4 out]
                    n168 = call "数值二进制转十进制-8.6.vi"("子数组"=w462) -> ("十进制数值"=w463:i32)  [unwired: 4 out]
                    n169 = call "数值二进制转十进制-8.6.vi"("子数组"=w448) -> ("十进制数值"=w449:i32)  [unwired: 4 out]
                    n170 = case shown="1" w463 {
                      tunnel: ["不公开" "公开"] -> w437
                      frame 0, Default {
                      }
                      frame 1 {
                      }
                    }
                    n171 = case shown="0, 默认" w459 {
                      tunnel: ["500Kps" "250Kps"] -> w438
                      frame 0, Default {
                      }
                      frame 1 {
                      }
                    }
                    n172 = Number To Decimal String(number=w449) -> (decimal integer string=w451:string)  [unwired: 1 out]
                    n173 = case shown="4" w460 {
                      tunnel: [_ "纯电动BMS" "混合动力BMS" "储能" "快换"] -> w439
                      frame 0, Default {
                      }
                      frame 1 {
                      }
                      frame 2 {
                      }
                      frame 3 {
                      }
                      frame 4 {
                      }
                    }
                    n174 = Number To Decimal String(number=w450) -> (decimal integer string=w453:string)  [unwired: 1 out]
                    n175 = call "运行模式解析.vi"("输入值"=w443) -> ("输出值"=w436:string)  [unwired: 1 in]
                    n176 = Concatenate Strings("V" ("字符串"), w451, "." ("字符串"), w453) -> (w440:string)
                    n177 = local read "高压板监控"() -> (w441:T10)
                    n178 = Bundle By Name(cluster=w441, "版本协议号"=w440, "应用类型"=w439, "波特率"=w438, "协议是否公开"=w437, "电池运行情况"=w436) -> (w435:T10)
                    n179 = local write "高压板监控"(w435) -> ()
                  }
                }
              }
            }
          }
          frame Error {
            n180 = Wait Until Next ms Multiple(millisecond multiple=u32 100 ("毫秒倍数")) -> ()  [unwired: 1 out]
          }
        }
      }
    }
    frame Enabled {
    }
  }
  n181 = while {
    shift-right: [w476] -> _
    shift-left: w50 -> [w475]
    shift-left: w50 -> [w474]
    stop <- w477 stop-if-true
    n182 = event shown="[0] 超时" {
      selector: _ -> [_ _ _ _]
      dyn-events: _ -> [_ _ _ _]
      timeout: 200 -> [_ _ _ _]
      tunnel: [_ _ _ w564] -> w477
      tunnel: [w482 w545 w556 w563] -> w476
      tunnel: w475 -> [w481 w545 w556 w563]
      tunnel: w474 -> [w480 _ _ _]
      event Timeout {
        n183 = event-data() -> ()  [unwired: 3 out]
        n184 = control-ref of="单选选项2 2"() -> (w484:refnum<vi>)
        n185 = control-ref of="单选选项2"() -> (w491:refnum<vi>)
        n186 = control-ref of="单选选项1"() -> (w492:refnum<vi>)
        n187 = local read "主界面选项"() -> (w493:enum32{"单选选项1", "单选选项2", "单选选项2 2"})
        n188 = Not Equal?(x=w481, y=w480) -> (x != y?=w479:bool)
        n189 = Build Array(w492, w491, w484) -> (w490:refnum<vi>[])
        n190 = local write "状态"(w479) -> ()
        n191 = case shown="\"单选选项1\", 默认" w493 {
          selector: w493 -> [w528 w535 w541]
          tunnel: w490 -> [w529 w538 w544]
          tunnel: [w527 w537 w543] -> w487
          tunnel: [w526 w536 w542] -> w486
          tunnel: [TRUE TRUE TRUE] -> w485
          tunnel: [enum32{"从板监控", "从板信息2", "电压温度", "高压板监控"}."从板监控" ("选项卡控件") enum32{"从板监控", "从板信息2", "电压温度", "高压板监控"}."从板信息2" ("选项卡控件") enum32{"从板监控", "从板信息2", "电压温度", "高压板监控"}."电压温度" ("选项卡控件")] -> w483
          frame "单选选项1", Default {
            n192 = local read "继电器状态"() -> (w532:string[])
            n193 = local read "快换帧"() -> (w531:T5)
            n194 = local read "最高电压位置"() -> (w507:i32)
            n195 = local read "最低电压位置"() -> (w506:i32)
            n196 = local read "最高温度位置"() -> (w503:i32)
            n197 = local read "最低温度位置"() -> (w502:i32)
            n198 = local read "最大内阻位置"() -> (w500:i32)
            n199 = local read "最小内阻位置"() -> (w498:i32)
            n200 = local read "最高电压"() -> (w509:dbl)
            n201 = local read "最低电压"() -> (w508:dbl)
            n202 = local read "最高温度"() -> (w505:dbl)
            n203 = local read "最低温度"() -> (w504:dbl)
            n204 = local read "最大内阻"() -> (w501:dbl)
            n205 = local read "最小内阻"() -> (w499:dbl)
            n206 = local read "故障信息"() -> (w511:string)
            n207 = Index Array(array=w532) -> (element #1=w520:string, element #2=w519:string, element #3=w518:string, element #4=w517:string, element #5=w516:string, element #6=w515:string, element #7=w514:string, element #8=w513:string)  [unwired: 8 in]
            n208 = Unbundle(w531) -> ("SOH"=w496:dbl, "充电总安时"=w524:dbl, "最大充电电流"=w523:dbl, "最大充电总电压"=w522:dbl)
            n209 = Delete From Array(array=w529, index=w528) -> (deleted portion=w526:refnum<vi>, array with subset deleted=w527:refnum<vi>[])  [unwired: 1 in]
            n210 = local read "从板参数"() -> (w521:T8)
            n211 = Subtract(x=w509, y=w508) -> (x-y=w510:dbl)
            n212 = Subtract(x=w505, y=w504) -> (x-y=w525:dbl)
            n213 = Bundle(cluster=w521, "最高电压"=w509, "位置1"=w507, "最低电压"=w508, "位置2"=w506, "压差"=w510, "最高温度"=w505, "位置3"=w503, "最低温度"=w504, "位置4"=w502, "温差"=w525, "最高内阻"=w501, "位置5"=w500, "最低内阻"=w499, "位置6"=w498, "故障信息"=w511, "最大充电总电压"=w522, "最大充电电流"=w523, "充电总安时"=w524, "SOH 2"=w496, "RL1_ST(fan)"=w520, "RL2_ST(heat)"=w519, "RL3_ST"=w518, "RL4_ST"=w517, "RL5_ST"=w516, "RL6_ST"=w515, "RL7_ST"=w514, "RL8_ST"=w513) -> (w530:T8)
            n214 = local write "从板参数"(w530) -> ()
          }
          frame "单选选项2" {
            n215 = Delete From Array(array=w538, index=w535) -> (deleted portion=w536:refnum<vi>, array with subset deleted=w537:refnum<vi>[])  [unwired: 1 in]
          }
          frame "单选选项2 2" {
            n216 = Delete From Array(array=w544, index=w541) -> (deleted portion=w542:refnum<vi>, array with subset deleted=w543:refnum<vi>[])  [unwired: 1 in]
          }
        }
        n217 = for {
          tunnel: w487 -> [w495] mode=indexing
          tunnel: u32 16777215 -> [w494]
          n218 = property class="Bool (严格)"(reference=w495, "BoolText.TextColor"=w494) -> ()  [unwired: 1 in, 2 out]
        }
        n219 = property class="Bool (严格)"(reference=w486, "BoolText.TextColor"=u32 65511) -> ()  [unwired: 1 in, 2 out]
        n220 = local write "选项卡控件"(w483) -> ()
        n221 = property on="从板板号 2" class="DigNum (严格)"("Visible"=w485) -> ()  [unwired: 2 in, 2 out]
        n222 = local read "Life:"() -> (w482:dbl)
      }
      event "从板板号 2": Value Change {
        n223 = event-data() -> ("OldVal"=w548:u8, "NewVal"=w547:u8)  [unwired: 5 out]
        n224 = Not Equal?(x=w548, y=w547) -> (x != y?=w546:bool)
        n225 = case shown="真" w546 {
          frame False {
          }
          frame True {
            w549 = 0
            w551 = T9 {"第1串"=0.0, "第2串"=0.0, "第3串"=0.0, "第4串"=0.0, "第5串"=0.0, "第6串"=0.0, "第7串"=0.0, "第8串"=0.0, "第9串"=0.0, "第10串"=0.0, "第11串"=0.0, "第12串"=0.0} ("1 102")
            w553 = 0.0 ("总电压")
            w554 = "" ("协议是否公开")
            n226 = local write "硬件故障"(string[][] [] ("电池故障 2")) -> ()
            n227 = local write "总电压(V)"(w553) -> ()
            n228 = local write "总电流(A)"(w553) -> ()
            n229 = local write "外总压(V)"(w553) -> ()
            n230 = local write "平均电流(A)"(w553) -> ()
            n231 = local write "SOH"(w553) -> ()
            n232 = local write "波特率"(w554) -> ()
            n233 = local write "滑动杆"(w553) -> ()
            n234 = local write "应用类型"(w554) -> ()
            n235 = local write "协议版本号"(w554) -> ()
            n236 = local write "协议是否公开"(w554) -> ()
            n237 = local write "电池充满标志位"(w554) -> ()
            n238 = local write "电池运行状态"(w554) -> ()
            n239 = local write "从板参数"(T12 {0.0, 0.0, 0.0, 0.0, 0.0, 0.0, 0.0, 0.0, 0.0, 0.0, 0.0, 0.0, 0.0, 0.0, "故障信息"="00", 0.0, 0.0, 0.0, 0.0, "RL1_ST"="", "RL2_ST"="", "RL3_ST"="", "RL4_ST"="", "RL5_ST"="", "RL6_ST"="", "RL7_ST"="", "RL8_ST"=""} ("从板参数")) -> ()
            n240 = local write "内部EE存储器状态"(w549) -> ()
            n241 = local write "系统时钟状态"(w549) -> ()
            n242 = local write "外部EE存储器状态"(w549) -> ()
            n243 = local write "供电电源状态"(w549) -> ()
            n244 = local write "温度模块检测状态"(w549) -> ()
            n245 = local write "电压模块检测状态"(w549) -> ()
            n246 = local write "绝缘检测模块状态"(w549) -> ()
            n247 = local write "电流模块模块状态"(w549) -> ()
            n248 = local write "内部总电压检测模块状态"(w549) -> ()
            n249 = local write "外部总电压检测模块状态"(w549) -> ()
            n250 = local write "电池放电均衡模块状态"(w549) -> ()
            n251 = local write "电池充电均衡模块状态"(w549) -> ()
            n252 = local write "1 102"(w551) -> ()
            n253 = local write "1"(w551) -> ()
            n254 = local write "2"(w551) -> ()
            n255 = local write "3"(w551) -> ()
            n256 = local write "4"(w551) -> ()
            n257 = local write "5"(w551) -> ()
            n258 = local write "Flash存储器状态"(w549) -> ()
            n259 = local write "1 3"(w551) -> ()
            n260 = local write "1 4"(w551) -> ()
            n261 = local write "1 6"(w551) -> ()
            n262 = local write "1 7"(w551) -> ()
          }
        }
      }
      event "刷新": Value Change {
        n263 = event-data() -> ("NewVal"=w555:bool)  [unwired: 6 out]
        n264 = case shown="真" w555 {
          frame False {
          }
          frame True {
            w557 = 0
            w559 = T9 {"第1串"=0.0, "第2串"=0.0, "第3串"=0.0, "第4串"=0.0, "第5串"=0.0, "第6串"=0.0, "第7串"=0.0, "第8串"=0.0, "第9串"=0.0, "第10串"=0.0, "第11串"=0.0, "第12串"=0.0} ("1 102")
            w561 = 0.0 ("总电压")
            w562 = "" ("协议是否公开")
            n265 = local write "硬件故障"(string[][] [] ("电池故障 2")) -> ()
            n266 = local write "总电压(V)"(w561) -> ()
            n267 = local write "总电流(A)"(w561) -> ()
            n268 = local write "外总压(V)"(w561) -> ()
            n269 = local write "平均电流(A)"(w561) -> ()
            n270 = local write "SOH"(w561) -> ()
            n271 = local write "波特率"(w562) -> ()
            n272 = local write "滑动杆"(w561) -> ()
            n273 = local write "应用类型"(w562) -> ()
            n274 = local write "协议版本号"(w562) -> ()
            n275 = local write "协议是否公开"(w562) -> ()
            n276 = local write "电池充满标志位"(w562) -> ()
            n277 = local write "电池运行状态"(w562) -> ()
            n278 = local write "从板参数"(T12 {0.0, 0.0, 0.0, 0.0, 0.0, 0.0, 0.0, 0.0, 0.0, 0.0, 0.0, 0.0, 0.0, 0.0, "故障信息"="00", 0.0, 0.0, 0.0, 0.0, "RL1_ST"="", "RL2_ST"="", "RL3_ST"="", "RL4_ST"="", "RL5_ST"="", "RL6_ST"="", "RL7_ST"="", "RL8_ST"=""} ("从板参数")) -> ()
            n279 = local write "内部EE存储器状态"(w557) -> ()
            n280 = local write "系统时钟状态"(w557) -> ()
            n281 = local write "外部EE存储器状态"(w557) -> ()
            n282 = local write "供电电源状态"(w557) -> ()
            n283 = local write "温度模块检测状态"(w557) -> ()
            n284 = local write "电压模块检测状态"(w557) -> ()
            n285 = local write "绝缘检测模块状态"(w557) -> ()
            n286 = local write "电流模块模块状态"(w557) -> ()
            n287 = local write "内部总电压检测模块状态"(w557) -> ()
            n288 = local write "外部总电压检测模块状态"(w557) -> ()
            n289 = local write "电池放电均衡模块状态"(w557) -> ()
            n290 = local write "电池充电均衡模块状态"(w557) -> ()
            n291 = local write "1 102"(w559) -> ()
            n292 = local write "1"(w559) -> ()
            n293 = local write "2"(w559) -> ()
            n294 = local write "3"(w559) -> ()
            n295 = local write "4"(w559) -> ()
            n296 = local write "5"(w559) -> ()
            n297 = local write "Flash存储器状态"(w557) -> ()
            n298 = local write "1 3"(w559) -> ()
            n299 = local write "1 4"(w559) -> ()
            n300 = local write "1 6"(w559) -> ()
            n301 = local write "1 7"(w559) -> ()
          }
        }
      }
      event Panel Close? {
        w564 = TRUE ("停止")
        n302 = event-data() -> ()  [unwired: 5 out]
        n303 = property class="VI"("FP.State"=T13."Hidden" ("前面板窗口:状态")) -> (reference out=w566:refnum<vi>, error out=w565:errorcluster)  [unwired: 2 in]
        n304 = local write "停止"(w564) -> ()
        n305 = property class="VI"(reference=w566, error in=w565, "Front Panel.Open"=FALSE ("前面板窗口:打开")) -> ()  [unwired: 2 out]
        n306 = event-data("Discard?"=w564) -> ()  [unwired: 1 in, 1 out]
      }
    }
    n307 = local write "状态"(FALSE ("状态")) -> ()
  }
  n308 = global read "功能码全局.vi" "14"() -> (w49:bool[])
  n309 = Index Array(array=w49, index=7 ("索引")) -> (element=w47:bool)
  n310 = property on="协议版本号" class="Str"("Visible"=w47) -> ()  [unwired: 2 in, 2 out]
  n311 = property on="波特率" class="Str"("Visible"=w47) -> ()  [unwired: 2 in, 2 out]
  n312 = property on="应用类型" class="Str"("Visible"=w47) -> ()  [unwired: 2 in, 2 out]
  n313 = property on="协议是否公开" class="Str"("Visible"=w47) -> ()  [unwired: 2 in, 2 out]
  n314 = call "自适应屏幕分辨率.vi"() -> ()  [unwired: 16 in]
  n315 = local write "停止"(FALSE ("停止")) -> ()
  n316 = global read "中英文全局.vi" "中英文选择"() -> (w46:enum32{"中文", "English"})
  n317 = while {
    stop <- w572 stop-if-true
    n318 = local read "从板板号 2"() -> (w571:u8)
    n319 = local read "布尔 2"() -> (w569:bool)
    n320 = local read "布尔"() -> (w570:bool)
    n321 = case shown="假" w569 {
      tunnel: w571 -> [_ w621]
      frame False {
        n322 = local read "布尔 3"() -> (w574:bool)
        n323 = case shown="真" w574 {
          frame False {
          }
          frame True {
            n324 = for {
              N: 5 -> [_]
              tunnel: bool[] [FALSE, FALSE, FALSE, FALSE, FALSE, FALSE, FALSE, FALSE, FALSE, FALSE, FALSE, FALSE, FALSE, FALSE, FALSE, FALSE, FALSE, FALSE, FALSE, FALSE, FALSE, FALSE, FALSE, FALSE, FALSE, FALSE, FALSE, FALSE, FALSE, FALSE, FALSE, FALSE, FALSE, FALSE, FALSE, FALSE, FALSE, FALSE, FALSE, FALSE, FALSE, FALSE, FALSE, FALSE, FALSE, FALSE, FALSE, FALSE, FALSE, FALSE, FALSE, FALSE, FALSE, FALSE, FALSE, FALSE, FALSE, FALSE, FALSE, FALSE] -> [w580]
              i -> [w579]
              w581 = 12 ("y")
              n325 = Multiply(x=w579, y=w581) -> (x*y=w582:i32)
              n326 = Array Subset(array=w580, index=w582, length=w581) -> (w578:bool[])
              n327 = case shown="4" w579 {
                tunnel: w578 -> [w584 w591 w598 w605 w612]
                frame 0, Default {
                  n328 = control-ref of="1"() -> (w583:refnum<vi>)
                  n329 = property class="Clust (严格)"(reference=w583) -> ("Controls[]"=w585:refnum<vi>[])  [unwired: 1 in, 2 out]
                  n330 = for {
                    tunnel: w585 -> [w588] mode=indexing
                    tunnel: w584 -> [w589]
                    i -> [w586]
                    n331 = Index Array(array=w589, index=w586) -> (element=w587:bool)
                    n332 = property class="Ctl"(reference=w588, "Blinking"=w587) -> ()  [unwired: 1 in, 2 out]
                  }
                }
                frame 1 {
                  n333 = control-ref of="2"() -> (w590:refnum<vi>)
                  n334 = property class="Clust (严格)"(reference=w590) -> ("Controls[]"=w592:refnum<vi>[])  [unwired: 1 in, 2 out]
                  n335 = for {
                    tunnel: w592 -> [w595] mode=indexing
                    tunnel: w591 -> [w596]
                    i -> [w593]
                    n336 = Index Array(array=w596, index=w593) -> (element=w594:bool)
                    n337 = property class="Ctl"(reference=w595, "Blinking"=w594) -> ()  [unwired: 1 in, 2 out]
                  }
                }
                frame 2 {
                  n338 = control-ref of="3"() -> (w597:refnum<vi>)
                  n339 = property class="Clust (严格)"(reference=w597) -> ("Controls[]"=w599:refnum<vi>[])  [unwired: 1 in, 2 out]
                  n340 = for {
                    tunnel: w599 -> [w602] mode=indexing
                    tunnel: w598 -> [w603]
                    i -> [w600]
                    n341 = Index Array(array=w603, index=w600) -> (element=w601:bool)
                    n342 = property class="Ctl"(reference=w602, "Blinking"=w601) -> ()  [unwired: 1 in, 2 out]
                  }
                }
                frame 3 {
                  n343 = control-ref of="4"() -> (w604:refnum<vi>)
                  n344 = property class="Clust (严格)"(reference=w604) -> ("Controls[]"=w606:refnum<vi>[])  [unwired: 1 in, 2 out]
                  n345 = for {
                    tunnel: w606 -> [w609] mode=indexing
                    tunnel: w605 -> [w610]
                    i -> [w607]
                    n346 = Index Array(array=w610, index=w607) -> (element=w608:bool)
                    n347 = property class="Ctl"(reference=w609, "Blinking"=w608) -> ()  [unwired: 1 in, 2 out]
                  }
                }
                frame 4 {
                  n348 = control-ref of="5"() -> (w611:refnum<vi>)
                  n349 = property class="Clust (严格)"(reference=w611) -> ("Controls[]"=w613:refnum<vi>[])  [unwired: 1 in, 2 out]
                  n350 = for {
                    tunnel: w613 -> [w616] mode=indexing
                    tunnel: w612 -> [w617]
                    i -> [w614]
                    n351 = Index Array(array=w617, index=w614) -> (element=w615:bool)
                    n352 = property class="Ctl"(reference=w616, "Blinking"=w615) -> ()  [unwired: 1 in, 2 out]
                  }
                }
              }
            }
            n353 = local write "布尔 3"(FALSE ("布尔 3")) -> ()
          }
        }
      }
      frame True {
        n354 = global read "单体信息全局.vi" "位置 2"() -> (w622:i32[])
        n355 = while {
          tunnel: w622 -> [w684]
          tunnel: w621 -> [w683]
          shift-right: [w680] -> _
          shift-left: 0 ("index of element") -> [w679]
          tunnel: [w678] -> w626 mode=indexing
          tunnel: [w677] -> w625
          i -> [w677]
          stop <- w681 stop-if-true
          n356 = Search 1D Array(1D array=w684, element=w683, start index (0)=w679) -> (index of element=w678:i32)
          n357 = Equal?(x=w678, y=-1) -> (x = y?=w681:bool)
          n358 = Increment(x=w678) -> (x+1=w680:i32)
        }
        n359 = global read "单体信息全局.vi" "数据 2"() -> (w624:dbl[])
        n360 = Reshape Array(w626, w625) -> (w627:i32[])
        n361 = for {
          tunnel: w624 -> [w676]
          tunnel: w627 -> [w675] mode=indexing
          tunnel: [w668] -> w619 mode=indexing
          n362 = local read "温度基准"() -> (w671:dbl)
          n363 = local read "偏差"() -> (w670:dbl)
          n364 = Index Array(array=w676, index=w675) -> (element=w672:dbl)
          n365 = Add(x=w671, y=w670) -> (x+y=w673:dbl)
          n366 = Subtract(x=w671, y=w670) -> (x-y=w674:dbl)
          n367 = In Range and Coerce(upper limit=w673, x=w672, lower limit=w674) -> (In Range?=w669:bool)  [unwired: 1 out]
          n368 = Not(x=w669) -> (.not. x?=w668:bool)
        }
        n369 = for {
          N: 5 -> [_]
          tunnel: w619 -> [w630]
          i -> [w629]
          w631 = 12 ("y")
          n370 = Multiply(x=w629, y=w631) -> (x*y=w632:i32)
          n371 = Array Subset(array=w630, index=w632, length=w631) -> (w628:bool[])
          n372 = case shown="2" w629 {
            tunnel: w628 -> [w634 w641 w648 w655 w662]
            frame 0, Default {
              n373 = control-ref of="1"() -> (w633:refnum<vi>)
              n374 = property class="Clust (严格)"(reference=w633) -> ("Controls[]"=w635:refnum<vi>[])  [unwired: 1 in, 2 out]
              n375 = for {
                tunnel: w635 -> [w638] mode=indexing
                tunnel: w634 -> [w639]
                i -> [w636]
                n376 = Index Array(array=w639, index=w636) -> (element=w637:bool)
                n377 = property class="Ctl"(reference=w638, "Blinking"=w637) -> ()  [unwired: 1 in, 2 out]
              }
            }
            frame 1 {
              n378 = control-ref of="2"() -> (w640:refnum<vi>)
              n379 = property class="Clust (严格)"(reference=w640) -> ("Controls[]"=w642:refnum<vi>[])  [unwired: 1 in, 2 out]
              n380 = for {
                tunnel: w642 -> [w645] mode=indexing
                tunnel: w641 -> [w646]
                i -> [w643]
                n381 = Index Array(array=w646, index=w643) -> (element=w644:bool)
                n382 = property class="Ctl"(reference=w645, "Blinking"=w644) -> ()  [unwired: 1 in, 2 out]
              }
            }
            frame 2 {
              n383 = control-ref of="3"() -> (w647:refnum<vi>)
              n384 = property class="Clust (严格)"(reference=w647) -> ("Controls[]"=w649:refnum<vi>[])  [unwired: 1 in, 2 out]
              n385 = for {
                tunnel: w649 -> [w652] mode=indexing
                tunnel: w648 -> [w653]
                i -> [w650]
                n386 = Index Array(array=w653, index=w650) -> (element=w651:bool)
                n387 = property class="Ctl"(reference=w652, "Blinking"=w651) -> ()  [unwired: 1 in, 2 out]
              }
            }
            frame 3 {
              n388 = control-ref of="4"() -> (w654:refnum<vi>)
              n389 = property class="Clust (严格)"(reference=w654) -> ("Controls[]"=w656:refnum<vi>[])  [unwired: 1 in, 2 out]
              n390 = for {
                tunnel: w656 -> [w659] mode=indexing
                tunnel: w655 -> [w660]
                i -> [w657]
                n391 = Index Array(array=w660, index=w657) -> (element=w658:bool)
                n392 = property class="Ctl"(reference=w659, "Blinking"=w658) -> ()  [unwired: 1 in, 2 out]
              }
            }
            frame 4 {
              n393 = control-ref of="5"() -> (w661:refnum<vi>)
              n394 = property class="Clust (严格)"(reference=w661) -> ("Controls[]"=w663:refnum<vi>[])  [unwired: 1 in, 2 out]
              n395 = for {
                tunnel: w663 -> [w666] mode=indexing
                tunnel: w662 -> [w667]
                i -> [w664]
                n396 = Index Array(array=w667, index=w664) -> (element=w665:bool)
                n397 = property class="Ctl"(reference=w666, "Blinking"=w665) -> ()  [unwired: 1 in, 2 out]
              }
            }
          }
        }
        n398 = local write "布尔 3"(TRUE ("布尔 3")) -> ()
      }
    }
    n399 = case shown="假" w570 {
      tunnel: w571 -> [_ w732]
      frame False {
        n400 = local read "布尔 3"() -> (w685:bool)
        n401 = case shown="真" w685 {
          frame False {
          }
          frame True {
            n402 = local write "布尔 3"(FALSE ("布尔 3")) -> ()
            n403 = for {
              N: 5 -> [_]
              tunnel: bool[] [FALSE, FALSE, FALSE, FALSE, FALSE, FALSE, FALSE, FALSE, FALSE, FALSE, FALSE, FALSE, FALSE, FALSE, FALSE, FALSE, FALSE, FALSE, FALSE, FALSE, FALSE, FALSE, FALSE, FALSE, FALSE, FALSE, FALSE, FALSE, FALSE, FALSE, FALSE, FALSE, FALSE, FALSE, FALSE, FALSE, FALSE, FALSE, FALSE, FALSE, FALSE, FALSE, FALSE, FALSE, FALSE, FALSE, FALSE, FALSE, FALSE, FALSE, FALSE, FALSE, FALSE, FALSE, FALSE, FALSE, FALSE, FALSE, FALSE, FALSE] -> [w691]
              i -> [w690]
              w692 = 12 ("y")
              n404 = Multiply(x=w690, y=w692) -> (x*y=w693:i32)
              n405 = Array Subset(array=w691, index=w693, length=w692) -> (w689:bool[])
              n406 = case shown="0, 默认" w690 {
                tunnel: w689 -> [w695 w702 w709 w716 w723]
                frame 0, Default {
                  n407 = control-ref of="1 102"() -> (w694:refnum<vi>)
                  n408 = property class="Clust (严格)"(reference=w694) -> ("Controls[]"=w696:refnum<vi>[])  [unwired: 1 in, 2 out]
                  n409 = for {
                    tunnel: w696 -> [w700] mode=indexing
                    tunnel: w695 -> [w699]
                    i -> [w698]
                    n410 = Index Array(array=w699, index=w698) -> (element=w697:bool)
                    n411 = property class="Ctl"(reference=w700, "Blinking"=w697) -> ()  [unwired: 1 in, 2 out]
                  }
                }
                frame 1 {
                  n412 = control-ref of="1 3"() -> (w701:refnum<vi>)
                  n413 = property class="Clust (严格)"(reference=w701) -> ("Controls[]"=w703:refnum<vi>[])  [unwired: 1 in, 2 out]
                  n414 = for {
                    tunnel: w703 -> [w706] mode=indexing
                    tunnel: w702 -> [w707]
                    i -> [w704]
                    n415 = Index Array(array=w707, index=w704) -> (element=w705:bool)
                    n416 = property class="Ctl"(reference=w706, "Blinking"=w705) -> ()  [unwired: 1 in, 2 out]
                  }
                }
                frame 2 {
                  n417 = control-ref of="1 4"() -> (w708:refnum<vi>)
                  n418 = property class="Clust (严格)"(reference=w708) -> ("Controls[]"=w710:refnum<vi>[])  [unwired: 1 in, 2 out]
                  n419 = for {
                    tunnel: w710 -> [w713] mode=indexing
                    tunnel: w709 -> [w714]
                    i -> [w711]
                    n420 = Index Array(array=w714, index=w711) -> (element=w712:bool)
                    n421 = property class="Ctl"(reference=w713, "Blinking"=w712) -> ()  [unwired: 1 in, 2 out]
                  }
                }
                frame 3 {
                  n422 = control-ref of="1 6"() -> (w715:refnum<vi>)
                  n423 = property class="Clust (严格)"(reference=w715) -> ("Controls[]"=w717:refnum<vi>[])  [unwired: 1 in, 2 out]
                  n424 = for {
                    tunnel: w717 -> [w720] mode=indexing
                    tunnel: w716 -> [w721]
                    i -> [w718]
                    n425 = Index Array(array=w721, index=w718) -> (element=w719:bool)
                    n426 = property class="Ctl"(reference=w720, "Blinking"=w719) -> ()  [unwired: 1 in, 2 out]
                  }
                }
                frame 4 {
                  n427 = control-ref of="1 7"() -> (w722:refnum<vi>)
                  n428 = property class="Clust (严格)"(reference=w722) -> ("Controls[]"=w724:refnum<vi>[])  [unwired: 1 in, 2 out]
                  n429 = for {
                    tunnel: w724 -> [w727] mode=indexing
                    tunnel: w723 -> [w728]
                    i -> [w725]
                    n430 = Index Array(array=w728, index=w725) -> (element=w726:bool)
                    n431 = property class="Ctl"(reference=w727, "Blinking"=w726) -> ()  [unwired: 1 in, 2 out]
                  }
                }
              }
            }
          }
        }
      }
      frame True {
        n432 = global read "单体信息全局.vi" "位置"() -> (w738:i32[])
        n433 = while {
          tunnel: w738 -> [w795]
          tunnel: w732 -> [w794]
          shift-right: [w791] -> _
          shift-left: 0 ("index of element") -> [w790]
          tunnel: [w789] -> w734 mode=indexing
          tunnel: [w788] -> w735
          i -> [w788]
          stop <- w792 stop-if-true
          n434 = Search 1D Array(1D array=w795, element=w794, start index (0)=w790) -> (index of element=w789:i32)
          n435 = Equal?(x=w789, y=-1) -> (x = y?=w792:bool)
          n436 = Increment(x=w789) -> (x+1=w791:i32)
        }
        n437 = global read "单体信息全局.vi" "数据"() -> (w736:dbl[])
        n438 = Reshape Array(w734, w735) -> (w733:i32[])
        n439 = for {
          tunnel: w736 -> [w787]
          tunnel: w733 -> [w786] mode=indexing
          tunnel: [w779] -> w730 mode=indexing
          n440 = local read "电压基准"() -> (w784:dbl)
          n441 = local read "偏差"() -> (w783:dbl)
          n442 = Index Array(array=w787, index=w786) -> (element=w785:dbl)
          n443 = Add(x=w784, y=w783) -> (x+y=w782:dbl)
          n444 = Subtract(x=w784, y=w783) -> (x-y=w781:dbl)
          n445 = In Range and Coerce(upper limit=w782, x=w785, lower limit=w781) -> (In Range?=w780:bool)  [unwired: 1 out]
          n446 = Not(x=w780) -> (.not. x?=w779:bool)
        }
        n447 = local write "布尔 3"(TRUE ("布尔 3")) -> ()
        n448 = for {
          N: 5 -> [_]
          tunnel: w730 -> [w741]
          i -> [w740]
          w742 = 12 ("y")
          n449 = Multiply(x=w740, y=w742) -> (x*y=w743:i32)
          n450 = Array Subset(array=w741, index=w743, length=w742) -> (w739:bool[])
          n451 = case shown="1" w740 {
            tunnel: w739 -> [w745 w752 w759 w766 w773]
            frame 0, Default {
              n452 = control-ref of="1 102"() -> (w744:refnum<vi>)
              n453 = property class="Clust (严格)"(reference=w744) -> ("Controls[]"=w746:refnum<vi>[])  [unwired: 1 in, 2 out]
              n454 = for {
                tunnel: w746 -> [w750] mode=indexing
                tunnel: w745 -> [w749]
                i -> [w748]
                n455 = Index Array(array=w749, index=w748) -> (element=w747:bool)
                n456 = property class="Ctl"(reference=w750, "Blinking"=w747) -> ()  [unwired: 1 in, 2 out]
              }
            }
            frame 1 {
              n457 = control-ref of="1 3"() -> (w751:refnum<vi>)
              n458 = property class="Clust (严格)"(reference=w751) -> ("Controls[]"=w753:refnum<vi>[])  [unwired: 1 in, 2 out]
              n459 = for {
                tunnel: w753 -> [w756] mode=indexing
                tunnel: w752 -> [w757]
                i -> [w754]
                n460 = Index Array(array=w757, index=w754) -> (element=w755:bool)
                n461 = property class="Ctl"(reference=w756, "Blinking"=w755) -> ()  [unwired: 1 in, 2 out]
              }
            }
            frame 2 {
              n462 = control-ref of="1 4"() -> (w758:refnum<vi>)
              n463 = property class="Clust (严格)"(reference=w758) -> ("Controls[]"=w760:refnum<vi>[])  [unwired: 1 in, 2 out]
              n464 = for {
                tunnel: w760 -> [w763] mode=indexing
                tunnel: w759 -> [w764]
                i -> [w761]
                n465 = Index Array(array=w764, index=w761) -> (element=w762:bool)
                n466 = property class="Ctl"(reference=w763, "Blinking"=w762) -> ()  [unwired: 1 in, 2 out]
              }
            }
            frame 3 {
              n467 = control-ref of="1 6"() -> (w765:refnum<vi>)
              n468 = property class="Clust (严格)"(reference=w765) -> ("Controls[]"=w767:refnum<vi>[])  [unwired: 1 in, 2 out]
              n469 = for {
                tunnel: w767 -> [w770] mode=indexing
                tunnel: w766 -> [w771]
                i -> [w768]
                n470 = Index Array(array=w771, index=w768) -> (element=w769:bool)
                n471 = property class="Ctl"(reference=w770, "Blinking"=w769) -> ()  [unwired: 1 in, 2 out]
              }
            }
            frame 4 {
              n472 = control-ref of="1 7"() -> (w772:refnum<vi>)
              n473 = property class="Clust (严格)"(reference=w772) -> ("Controls[]"=w774:refnum<vi>[])  [unwired: 1 in, 2 out]
              n474 = for {
                tunnel: w774 -> [w777] mode=indexing
                tunnel: w773 -> [w778]
                i -> [w775]
                n475 = Index Array(array=w778, index=w775) -> (element=w776:bool)
                n476 = property class="Ctl"(reference=w777, "Blinking"=w776) -> ()  [unwired: 1 in, 2 out]
              }
            }
          }
        }
      }
    }
    n477 = Wait Until Next ms Multiple(millisecond multiple=u32 1000 ("毫秒倍数")) -> ()  [unwired: 1 out]
    n478 = local read "停止"() -> (w572:bool)
  }
  n479 = while {
    stop <- w797 stop-if-true
    n480 = local read "选项卡控件"() -> (w796:enum32{"从板监控", "从板信息2", "电压温度", "高压板监控"})
    n481 = case shown="\"电压温度\"" w796 {
      frame "从板监控", Default {
      }
      frame "电压温度" {
        n482 = global read "单体信息全局.vi" "位置 2"() -> (w804:i32[])
        n483 = local read "从板板号 2"() -> (w803:u8)
        n484 = global read "单体信息全局.vi" "位置"() -> (w831:i32[])
        n485 = while {
          tunnel: w804 -> [w964]
          tunnel: w803 -> [w963]
          shift-right: [w960] -> _
          shift-left: 0 ("index of element") -> [w959]
          tunnel: [w958] -> w808 mode=indexing
          tunnel: [w957] -> w807
          i -> [w957]
          stop <- w961 stop-if-true
          n486 = Search 1D Array(1D array=w964, element=w963, start index (0)=w959) -> (index of element=w958:i32)
          n487 = Equal?(x=w958, y=-1) -> (x = y?=w961:bool)
          n488 = Increment(x=w958) -> (x+1=w960:i32)
        }
        n489 = while {
          tunnel: w831 -> [w987]
          tunnel: w803 -> [w986]
          shift-right: [w983] -> _
          shift-left: 0 ("index of element") -> [w982]
          tunnel: [w981] -> w827 mode=indexing
          tunnel: [w980] -> w828
          i -> [w980]
          stop <- w984 stop-if-true
          n490 = Search 1D Array(1D array=w987, element=w986, start index (0)=w982) -> (index of element=w981:i32)
          n491 = Equal?(x=w981, y=-1) -> (x = y?=w984:bool)
          n492 = Increment(x=w981) -> (x+1=w983:i32)
        }
        n493 = global read "单体信息全局.vi" "数据 2"() -> (w806:dbl[])
        n494 = global read "单体信息全局.vi" "数据"() -> (w829:dbl[])
        n495 = Reshape Array(w808, w807) -> (w809:i32[])
        n496 = Reshape Array(w827, w828) -> (w826:i32[])
        n497 = for {
          tunnel: w806 -> [w956]
          tunnel: w809 -> [w955] mode=indexing
          tunnel: [w954] -> w817 mode=indexing
          tunnel: [TRUE] -> w799 mode=indexing
          n498 = Index Array(array=w956, index=w955) -> (element=w954:dbl)
        }
        n499 = for {
          tunnel: w829 -> [w979]
          tunnel: w826 -> [w978] mode=indexing
          tunnel: [w977] -> w818 mode=indexing
          tunnel: [TRUE] -> w801 mode=indexing
          n500 = Index Array(array=w979, index=w978) -> (element=w977:dbl)
        }
        n501 = Array Size(array=w817) -> (size(s)=w815:i32)
        n502 = Array Size(array=w818) -> (size(s)=w820:i32)
        n503 = Quotient & Remainder(x=w815, y=12) -> (x-y*floor(x/y)=w811:i32, floor(x/y)=w813:i32)
        n504 = for {
          N: 5 -> [_]
          tunnel: w801 -> [w889]
          i -> [w888]
          w890 = 12 ("y")
          n505 = Multiply(x=w888, y=w890) -> (x*y=w891:i32)
          n506 = Array Subset(array=w889, index=w891, length=w890) -> (w887:bool[])
          n507 = case shown="4" w888 {
            tunnel: w887 -> [w893 w903 w913 w923 w933]
            frame 0, Default {
              n508 = control-ref of="1 102"() -> (w892:refnum<vi>)
              n509 = property class="Clust (严格)"(reference=w892) -> ("Controls[]"=w894:refnum<vi>[])  [unwired: 1 in, 2 out]
              n510 = for {
                tunnel: w894 -> [w901] mode=indexing
                tunnel: w893 -> [w900]
                i -> [w899]
                n511 = Index Array(array=w900, index=w899) -> (element=w898:bool)
                n512 = Select(t=0, s=w898, f=2) -> (s? t:f=w895:i32)
                n513 = property class="Ctl"(reference=w901, "DisabledEnum"=w895) -> ()  [unwired: 1 in, 2 out]
              }
            }
            frame 1 {
              n514 = control-ref of="1 3"() -> (w902:refnum<vi>)
              n515 = property class="Clust (严格)"(reference=w902) -> ("Controls[]"=w904:refnum<vi>[])  [unwired: 1 in, 2 out]
              n516 = for {
                tunnel: w904 -> [w910] mode=indexing
                tunnel: w903 -> [w911]
                i -> [w909]
                n517 = Index Array(array=w911, index=w909) -> (element=w906:bool)
                n518 = Select(t=0, s=w906, f=2) -> (s? t:f=w905:i32)
                n519 = property class="Ctl"(reference=w910, "DisabledEnum"=w905) -> ()  [unwired: 1 in, 2 out]
              }
            }
            frame 2 {
              n520 = control-ref of="1 4"() -> (w912:refnum<vi>)
              n521 = property class="Clust (严格)"(reference=w912) -> ("Controls[]"=w914:refnum<vi>[])  [unwired: 1 in, 2 out]
              n522 = for {
                tunnel: w914 -> [w920] mode=indexing
                tunnel: w913 -> [w921]
                i -> [w919]
                n523 = Index Array(array=w921, index=w919) -> (element=w916:bool)
                n524 = Select(t=0, s=w916, f=2) -> (s? t:f=w915:i32)
                n525 = property class="Ctl"(reference=w920, "DisabledEnum"=w915) -> ()  [unwired: 1 in, 2 out]
              }
            }
            frame 3 {
              n526 = control-ref of="1 6"() -> (w922:refnum<vi>)
              n527 = property class="Clust (严格)"(reference=w922) -> ("Controls[]"=w924:refnum<vi>[])  [unwired: 1 in, 2 out]
              n528 = for {
                tunnel: w924 -> [w930] mode=indexing
                tunnel: w923 -> [w931]
                i -> [w929]
                n529 = Index Array(array=w931, index=w929) -> (element=w926:bool)
                n530 = Select(t=0, s=w926, f=2) -> (s? t:f=w925:i32)
                n531 = property class="Ctl"(reference=w930, "DisabledEnum"=w925) -> ()  [unwired: 1 in, 2 out]
              }
            }
            frame 4 {
              n532 = control-ref of="1 7"() -> (w932:refnum<vi>)
              n533 = property class="Clust (严格)"(reference=w932) -> ("Controls[]"=w934:refnum<vi>[])  [unwired: 1 in, 2 out]
              n534 = for {
                tunnel: w934 -> [w940] mode=indexing
                tunnel: w933 -> [w941]
                i -> [w939]
                n535 = Index Array(array=w941, index=w939) -> (element=w936:bool)
                n536 = Select(t=0, s=w936, f=2) -> (s? t:f=w935:i32)
                n537 = property class="Ctl"(reference=w940, "DisabledEnum"=w935) -> ()  [unwired: 1 in, 2 out]
              }
            }
          }
        }
        n538 = Quotient & Remainder(x=w820, y=12) -> (x-y*floor(x/y)=w824:i32, floor(x/y)=w822:i32)
        n539 = Equal To 0?(x=w811) -> (x = 0?=w812:bool)
        n540 = for {
          N: 5 -> [_]
          tunnel: w799 -> [w834]
          i -> [w833]
          w835 = 12 ("y")
          n541 = Multiply(x=w833, y=w835) -> (x*y=w836:i32)
          n542 = Array Subset(array=w834, index=w836, length=w835) -> (w832:bool[])
          n543 = case shown="1" w833 {
            tunnel: w832 -> [w838 w848 w858 w868 w878]
            frame 0, Default {
              n544 = control-ref of="1"() -> (w837:refnum<vi>)
              n545 = property class="Clust (严格)"(reference=w837) -> ("Controls[]"=w839:refnum<vi>[])  [unwired: 1 in, 2 out]
              n546 = for {
                tunnel: w839 -> [w845] mode=indexing
                tunnel: w838 -> [w846]
                i -> [w844]
                n547 = Index Array(array=w846, index=w844) -> (element=w841:bool)
                n548 = Select(t=0, s=w841, f=2) -> (s? t:f=w840:i32)
                n549 = property class="Ctl"(reference=w845, "DisabledEnum"=w840) -> ()  [unwired: 1 in, 2 out]
              }
            }
            frame 1 {
              n550 = control-ref of="2"() -> (w847:refnum<vi>)
              n551 = property class="Clust (严格)"(reference=w847) -> ("Controls[]"=w849:refnum<vi>[])  [unwired: 1 in, 2 out]
              n552 = for {
                tunnel: w849 -> [w855] mode=indexing
                tunnel: w848 -> [w856]
                i -> [w854]
                n553 = Index Array(array=w856, index=w854) -> (element=w851:bool)
                n554 = Select(t=0, s=w851, f=2) -> (s? t:f=w850:i32)
                n555 = property class="Ctl"(reference=w855, "DisabledEnum"=w850) -> ()  [unwired: 1 in, 2 out]
              }
            }
            frame 2 {
              n556 = control-ref of="3"() -> (w857:refnum<vi>)
              n557 = property class="Clust (严格)"(reference=w857) -> ("Controls[]"=w859:refnum<vi>[])  [unwired: 1 in, 2 out]
              n558 = for {
                tunnel: w859 -> [w865] mode=indexing
                tunnel: w858 -> [w866]
                i -> [w864]
                n559 = Index Array(array=w866, index=w864) -> (element=w861:bool)
                n560 = Select(t=0, s=w861, f=2) -> (s? t:f=w860:i32)
                n561 = property class="Ctl"(reference=w865, "DisabledEnum"=w860) -> ()  [unwired: 1 in, 2 out]
              }
            }
            frame 3 {
              n562 = control-ref of="4"() -> (w867:refnum<vi>)
              n563 = property class="Clust (严格)"(reference=w867) -> ("Controls[]"=w869:refnum<vi>[])  [unwired: 1 in, 2 out]
              n564 = for {
                tunnel: w869 -> [w875] mode=indexing
                tunnel: w868 -> [w876]
                i -> [w874]
                n565 = Index Array(array=w876, index=w874) -> (element=w871:bool)
                n566 = Select(t=0, s=w871, f=2) -> (s? t:f=w870:i32)
                n567 = property class="Ctl"(reference=w875, "DisabledEnum"=w870) -> ()  [unwired: 1 in, 2 out]
              }
            }
            frame 4 {
              n568 = control-ref of="5"() -> (w877:refnum<vi>)
              n569 = property class="Clust (严格)"(reference=w877) -> ("Controls[]"=w879:refnum<vi>[])  [unwired: 1 in, 2 out]
              n570 = for {
                tunnel: w879 -> [w885] mode=indexing
                tunnel: w878 -> [w886]
                i -> [w884]
                n571 = Index Array(array=w886, index=w884) -> (element=w881:bool)
                n572 = Select(t=0, s=w881, f=2) -> (s? t:f=w880:i32)
                n573 = property class="Ctl"(reference=w885, "DisabledEnum"=w880) -> ()  [unwired: 1 in, 2 out]
              }
            }
          }
        }
        n574 = Equal To 0?(x=w824) -> (x = 0?=w823:bool)
        n575 = Increment(x=w813) -> (x+1=w814:i32)
        n576 = Increment(x=w822) -> (x+1=w821:i32)
        n577 = Select(t=w813, s=w812, f=w814) -> (s? t:f=w816:i32)
        n578 = Select(t=w822, s=w823, f=w821) -> (s? t:f=w819:i32)
        n579 = for {
          N: w816 -> [_]
          tunnel: w817 -> [w947]
          i -> [w944]
          w945 = 12 ("y")
          n580 = Multiply(x=w944, y=w945) -> (x*y=w946:i32)
          n581 = Array Subset(array=w947, index=w946, length=w945) -> (w943:dbl[])
          n582 = Array To Cluster(array=w943) -> (cluster=w942:T14)
          n583 = case shown="4" w944 {
            tunnel: w942 -> [w948 w949 w950 w951 w952]
            frame 0, Default {
              n584 = local write "1"(w948) -> ()
            }
            frame 1 {
              n585 = local write "2"(w949) -> ()
            }
            frame 2 {
              n586 = local write "3"(w950) -> ()
            }
            frame 3 {
              n587 = local write "4"(w951) -> ()
            }
            frame 4 {
              n588 = local write "5"(w952) -> ()
            }
          }
        }
        n589 = for {
          N: w819 -> [_]
          tunnel: w818 -> [w970]
          i -> [w967]
          w968 = 12 ("y")
          n590 = Multiply(x=w967, y=w968) -> (x*y=w969:i32)
          n591 = Array Subset(array=w970, index=w969, length=w968) -> (w966:dbl[])
          n592 = Array To Cluster(array=w966) -> (cluster=w965:T14)
          n593 = case shown="4" w967 {
            tunnel: w965 -> [w971 w972 w973 w974 w975]
            frame 0, Default {
              n594 = local write "1 102"(w971) -> ()
            }
            frame 1 {
              n595 = local write "1 3"(w972) -> ()
            }
            frame 2 {
              n596 = local write "1 4"(w973) -> ()
            }
            frame 3 {
              n597 = local write "1 6"(w974) -> ()
            }
            frame 4 {
              n598 = local write "1 7"(w975) -> ()
            }
          }
        }
      }
    }
    n599 = Wait Until Next ms Multiple(millisecond multiple=u32 500 ("毫秒倍数")) -> ()  [unwired: 1 out]
    n600 = local read "停止"() -> (w797:bool)
  }
  n601 = while {
    stop <- "停止" stop-if-true
    n602 = local read "从板板号 2"() -> (w1095:u8)
    n603 = global read "从板全局变量.vi" "最高电压位置"() -> (w1087:dbl[])
    n604 = global read "从板全局变量.vi" "最低电压位置"() -> (w1086:dbl[])
    n605 = global read "从板全局变量.vi" "最高温度位置"() -> (w1083:dbl[])
    n606 = global read "从板全局变量.vi" "最低温度位置"() -> (w1082:dbl[])
    n607 = global read "从板全局变量.vi" "平均电流"() -> (w1091:dbl[])
    n608 = global read "从板全局变量.vi" "最高电压"() -> (w1089:dbl[])
    n609 = global read "从板全局变量.vi" "最低电压"() -> (w1088:dbl[])
    n610 = global read "从板全局变量.vi" "最高温度"() -> (w1085:dbl[])
    n611 = global read "从板全局变量.vi" "最低温度"() -> (w1084:dbl[])
    n612 = global read "从板全局变量.vi" "总电压"() -> (w1096:dbl[])
    n613 = global read "从板全局变量.vi" "外总压"() -> (w1093:dbl[])
    n614 = global read "从板全局变量.vi" "总电流"() -> (w1090:dbl[])
    n615 = global read "从板全局变量.vi" "SOC"() -> (w1081:dbl[])
    n616 = global read "从板全局变量.vi" "SOH"() -> (w1080:dbl[])
    n617 = Decrement(x=w1095) -> (x-1=w994:u8)
    n618 = Index Array(array=w1096, index=w994) -> (element=w1094:dbl)
    n619 = Index Array(array=w1083, index=w994) -> (element=→"最高温度位置":dbl)
    n620 = Index Array(array=w1093, index=w994) -> (element=w1092:dbl)
    n621 = Index Array(array=w1091, index=w994) -> (element=w1079:dbl)
    n622 = Index Array(array=w1090, index=w994) -> (element=w1078:dbl)
    n623 = Index Array(array=w1086, index=w994) -> (element=→"最低电压位置":dbl)
    n624 = Index Array(array=w1085, index=w994) -> (element=→"最高温度":dbl)
    n625 = Index Array(array=w1080, index=w994) -> (element=w1068:dbl)
    n626 = Index Array(array=w1089, index=w994) -> (element=→"最高电压":dbl)
    n627 = Index Array(array=w1088, index=w994) -> (element=→"最低电压":dbl)
    n628 = Index Array(array=w1081, index=w994) -> (element=w1069:dbl)
    n629 = Index Array(array=w1084, index=w994) -> (element=→"最低温度":dbl)
    n630 = Index Array(array=w1087, index=w994) -> (element=→"最高电压位置":dbl)
    n631 = Index Array(array=w1082, index=w994) -> (element=→"最低温度位置":dbl)
    n632 = local write "总电压(V)"(w1094) -> ()
    n633 = local write "外总压(V)"(w1092) -> ()
    n634 = local write "总电流(A)"(w1078) -> ()
    n635 = local write "平均电流(A)"(w1079) -> ()
    n636 = local write "SOH"(w1068) -> ()
    n637 = local write "滑动杆"(w1069) -> ()
    n638 = global read "从板全局变量.vi" "最大内阻位置"() -> (w1056:dbl[])
    n639 = global read "从板全局变量.vi" "最小内阻位置"() -> (w1057:dbl[])
    n640 = global read "从板全局变量.vi" "协议是否公开"() -> (w1062:string[])
    n641 = global read "从板全局变量.vi" "电池运行状态"() -> (w1063:string[])
    n642 = global read "从板全局变量.vi" "最大内阻"() -> (w1054:dbl[])
    n643 = global read "从板全局变量.vi" "最小内阻"() -> (w1055:dbl[])
    n644 = global read "从板全局变量.vi" "故障信息"() -> (w1058:string[])
    n645 = global read "从板全局变量.vi" "应用类型"() -> (w1060:string[])
    n646 = global read "从板全局变量.vi" "继电器1"() -> (w1065:dbl[])
    n647 = global read "从板全局变量.vi" "继电器2"() -> (w1066:dbl[])
    n648 = global read "从板全局变量.vi" "版本号"() -> (w1059:string[])
    n649 = global read "从板全局变量.vi" "波特率"() -> (w1061:string[])
    n650 = global read "从板全局变量.vi" "满标志"() -> (w1067:dbl[])
    n651 = global read "从板全局变量.vi" "Life"() -> (w1064:dbl[])
    n652 = Index Array(array=w1054, index=w994) -> (element=→"最大内阻":dbl)
    n653 = Index Array(array=w1064, index=w994) -> (element=w991:dbl)
    n654 = Index Array(array=w1055, index=w994) -> (element=→"最小内阻":dbl)
    n655 = Index Array(array=w1056, index=w994) -> (element=→"最大内阻位置":dbl)
    n656 = Index Array(array=w1057, index=w994) -> (element=→"最小内阻位置":dbl)
    n657 = Index Array(array=w1061, index=w994) -> (element=w1051:string)
    n658 = Index Array(array=w1062, index=w994) -> (element=w1052:string)
    n659 = Index Array(array=w1065, index=w994) -> (element=w1043:dbl)
    n660 = Index Array(array=w1067, index=w994) -> (element=w1041:dbl)
    n661 = Index Array(array=w1058, index=w994) -> (element=→"故障信息":string)
    n662 = Index Array(array=w1059, index=w994) -> (element=w1049:string)
    n663 = Index Array(array=w1066, index=w994) -> (element=w1042:dbl)
    n664 = Index Array(array=w1063, index=w994) -> (element=w1053:string)
    n665 = Index Array(array=w1060, index=w994) -> (element=w1050:string)
    n666 = local write "协议版本号"(w1049) -> ()
    n667 = local write "波特率"(w1051) -> ()
    n668 = local write "应用类型"(w1050) -> ()
    n669 = local write "协议是否公开"(w1052) -> ()
    n670 = local write "电池运行状态"(w1053) -> ()
    n671 = local write "Life:"(w991) -> ()
    n672 = global read "中英文全局.vi" "中英文选择"() -> (w988:enum32{"中文", "English"})
    n673 = case shown="\"中文\"" w988 {
      tunnel: [w1110 w1115] -> w1107
      tunnel: w1041 -> [w1109 w1114]
      frame "English" {
        n674 = case shown="AA" w1109 {
          tunnel: [_ "Clean" "Charge,But not full" "Full"] -> w1110
          frame 0, Default {
          }
          frame 85 {
          }
          frame 90 {
          }
          frame 170 {
          }
        }
      }
      frame "中文" {
        n675 = case shown="5A" w1114 {
          tunnel: [_ "清除" "充电,但未充满" "充满"] -> w1115
          frame 0, Default {
          }
          frame 85 {
          }
          frame 90 {
          }
          frame 170 {
          }
        }
      }
    }
    n676 = call "各种状态子VI.vi"("颜色输入"=u32[] [16448250, 6618880, 16711680, 16860], "状态输入"=string[][] [["Close", "Open", "Fault", "Invalid"], ["Close", "Open", "Fault", "Invalid"], ["Close", "Open", "Fault", "Invalid"], ["Close", "Open", "Fault", "Invalid"]], "几种类型"=4, "数值"=w1043) -> ("状态"=w1104:string[])  [unwired: 1 out]
    n677 = call "各种状态子VI.vi"("颜色输入"=u32[] [16448250, 6618880, 16711680, 16860], "状态输入"=string[][] [["Close", "Open", "Fault", "Invalid"], ["Close", "Open", "Fault", "Invalid"], ["Close", "Open", "Fault", "Invalid"], ["Close", "Open", "Fault", "Invalid"]], "几种类型"=4, "数值"=w1042) -> ("状态"=w1105:string[])  [unwired: 1 out]
    n678 = local write "电池充满标志位"(w1107) -> ()
    n679 = Build Array(w1104, w1105) -> (w1106:string[][])
    n680 = Reshape Array(w1106, 8 ("维数大小")) -> (w989:string[])
    n681 = local write "继电器状态"(w989) -> ()
    n682 = global read "从板全局变量.vi" "F"() -> (w996:dbl[][])
    n683 = global read "从板全局变量.vi" "故障信息"() -> (w1028:string[])
    n684 = Index Array(array=w996, index (row)=w994) -> (element=w995:dbl[])  [unwired: 1 in]
    n685 = Index Array(array=w1028, index=w994) -> (element=w1026:string)
    n686 = Index Array(array=w995) -> (element #1=w1004:dbl, element #2=w1003:dbl, element #3=w1002:dbl, element #4=w1001:dbl, element #5=w999:dbl, element #6=w997:dbl)  [unwired: 6 in]
    n687 = for {
      N: 8 -> [_]
      tunnel: w1026 -> [w1164]
      tunnel: [w1159] -> w1025 mode=indexing
      i -> [w1163]
      w1161 = 2 ("x")
      n688 = Multiply(x=w1161, y=w1163) -> (x*y=w1162:i32)
      n689 = String Subset(string=w1164, offset (0)=w1162, length (rest)=w1161) -> (substring=w1160:string)
      n690 = Hexadecimal String To Number(string=w1160, default (0uL)=u8 0) -> (number=w1159:u8)  [unwired: 1 in, 1 out]
    }
    n691 = Format Into String(format string="%#f" ("格式字符串"), w997) -> (resulting string=→"供电电源电压(V)":string)  [unwired: 2 in, 1 out]
    n692 = Format Into String(format string="%#f" ("格式字符串"), w999) -> (resulting string=→"内网总线负载率":string)  [unwired: 2 in, 1 out]
    n693 = call "二进制解析-8.6.vi"("索引"=8, "数值"=w1003) -> ("低位子数组"=w1014:i32[])  [unwired: 3 out]
    n694 = call "二进制解析-8.6.vi"("索引"=8, "数值"=w1001) -> ("低位子数组"=w1007:i32[])  [unwired: 3 out]
    n695 = call "二进制解析-8.6.vi"("索引"=8, "数值"=w1004) -> ("低位子数组"=w1013:i32[])  [unwired: 3 out]
    n696 = call "二进制解析-8.6.vi"("索引"=8, "数值"=w1002) -> ("低位子数组"=w1008:i32[])  [unwired: 3 out]
    n697 = Index Array(array=w1025) -> (element #1=w1024:u8, element #2=w1023:u8, element #3=w1022:u8, element #4=w1021:u8, element #5=w1020:u8, element #6=w1019:u8, element #7=w1018:u8, element #8=w1017:u8)  [unwired: 8 in]
    n698 = for {
      N: 2 -> [_]
      tunnel: w1007 -> [w1124]
      i -> [w1122]
      w1126 = 2 ("y")
      n699 = Multiply(x=w1122, y=w1126) -> (x*y=w1125:i32)
      n700 = Array Subset(array=w1124, index=w1125, length=w1126) -> (w1123:i32[])
      n701 = call "数值二进制转十进制-8.6.vi"("子数组"=w1123) -> ("十进制数值"=w1121:i32)  [unwired: 4 out]
      n702 = case shown="1" w1122 {
        tunnel: w1121 -> [_ w1127 _ _]
        frame 0, Default {
        }
        frame 1 {
          "供电电源状态" <- w1127
        }
        frame 2 {
        }
        frame 3 {
        }
      }
    }
    n703 = for {
      N: 4 -> [_]
      tunnel: w1014 -> [w1141]
      i -> [w1139]
      w1143 = 2 ("y")
      n704 = Multiply(x=w1139, y=w1143) -> (x*y=w1142:i32)
      n705 = Array Subset(array=w1141, index=w1142, length=w1143) -> (w1140:i32[])
      n706 = call "数值二进制转十进制-8.6.vi"("子数组"=w1140) -> ("十进制数值"=w1138:i32)  [unwired: 4 out]
      n707 = case shown="3" w1139 {
        tunnel: w1138 -> [w1144 w1145 w1146 w1147]
        frame 0, Default {
          "绝缘检测模块状态" <- w1144
        }
        frame 1 {
          "电流模块模块状态" <- w1145
        }
        frame 2 {
          "电池充电均衡模块状态" <- w1146
        }
        frame 3 {
          "电池放电均衡模块状态" <- w1147
        }
      }
    }
    n708 = for {
      N: 4 -> [_]
      tunnel: w1013 -> [w1151]
      i -> [w1149]
      w1153 = 2 ("y")
      n709 = Multiply(x=w1149, y=w1153) -> (x*y=w1152:i32)
      n710 = Array Subset(array=w1151, index=w1152, length=w1153) -> (w1150:i32[])
      n711 = call "数值二进制转十进制-8.6.vi"("子数组"=w1150) -> ("十进制数值"=w1148:i32)  [unwired: 4 out]
      n712 = case shown="0, 默认" w1149 {
        tunnel: w1148 -> [w1154 w1155 w1156 w1157]
        frame 0, Default {
          "温度模块检测状态" <- w1154
        }
        frame 1 {
          "内部总电压检测模块状态" <- w1155
        }
        frame 2 {
          "外部总电压检测模块状态" <- w1156
        }
        frame 3 {
          "电压模块检测状态" <- w1157
        }
      }
    }
    n713 = for {
      N: 4 -> [_]
      tunnel: w1008 -> [w1131]
      i -> [w1129]
      w1133 = 2 ("y")
      n714 = Multiply(x=w1129, y=w1133) -> (x*y=w1132:i32)
      n715 = Array Subset(array=w1131, index=w1132, length=w1133) -> (w1130:i32[])
      n716 = call "数值二进制转十进制-8.6.vi"("子数组"=w1130) -> ("十进制数值"=w1128:i32)  [unwired: 4 out]
      n717 = case shown="2" w1129 {
        tunnel: w1128 -> [w1134 w1135 w1136 w1137]
        frame 0, Default {
          "系统时钟状态" <- w1134
        }
        frame 1 {
          "Flash存储器状态" <- w1135
        }
        frame 2 {
          "外部EE存储器状态" <- w1136
        }
        frame 3 {
          "内部EE存储器状态" <- w1137
        }
      }
    }
    n718 = call "故障数值解析.vi"("输入"=w1024) -> ("结果"=w1039:string[])  [unwired: 2 out]
    n719 = call "故障数值解析.vi"("输入"=w1023) -> ("结果"=w1038:string[])  [unwired: 2 out]
    n720 = call "故障数值解析.vi"("输入"=w1022) -> ("结果"=w1037:string[])  [unwired: 2 out]
    n721 = call "故障数值解析.vi"("输入"=w1021) -> ("结果"=w1033:string[])  [unwired: 2 out]
    n722 = call "故障数值解析.vi"("输入"=w1020) -> ("结果"=w1036:string[])  [unwired: 2 out]
    n723 = call "故障数值解析.vi"("输入"=w1019) -> ("结果"=w1035:string[])  [unwired: 2 out]
    n724 = call "故障数值解析.vi"("输入"=w1018) -> ("结果"=w1034:string[])  [unwired: 2 out]
    n725 = call "故障数值解析.vi"("输入"=w1017) -> ("结果"=w1032:string[])  [unwired: 2 out]
    n726 = Build Array(w1039, w1038, w1037, w1033, w1036, w1035, w1034, w1032) -> (w1030:string[][])
    n727 = Reshape Array(w1030, 32 ("维数大小")) -> (w1029:string[])
    n728 = case shown="\"English\"" w988 {
      tunnel: [string[] ["电压检测模块故障", "温度检测模块故障", "电流检测模块故障", "绝缘检测模块故障", "内总电压检测模块故障", "外总电压检测模块故障", "系统外扩时钟模块故障", "CPU内部EE故障", "EE存储器故障", "45db041存储器故障", "CPU内部FLASH存储器故障", "CPU故障", "CAN4通信模块故障", "CAN0通信模块故障", "CAN1通信模块故障", "保留", "保留", "保留", "保留", "保留", "充电均衡模块故障", "放电均衡模块故障", "保留", "软件故障", "保留", "保留", "保留", "保留", "DI模块故障", "DO模块故障", "保留", "保留"] ("名称") string[] ["detection_cellv", "detection_temper", "detection_curr", "detection_iso", "detection_sumv_in", "detection_sumv_out", "detection_exterm_clock", "detection_ee_cpu", "detection_ee_ext", "detection_flash_ext", "detection_flash_cpu", "cpu_error", "detection_can4", "detection_can0", "detection_can1", "rsv", "rsv", "rsv", "rsv", "rsv", "detection_chg_bal", "detection_dch_bal", "rsv", "soft_error", "rsv", "rsv", "rsv", "rsv", "DI_error", "DO_error", "rsv", "rsv"] ("名称")] -> w1040
      frame "中文", Default {
      }
      frame "English" {
      }
    }
    n729 = call "故障分解.vi"("名称"=w1040, "故障输入口"=w1029) -> ("输出数组"=→"硬件故障":string[][])  [unwired: 1 in, 2 out]
  }
  n730 = case shown="\"English\"" w46 {
    tunnel: ["总电压(V)" "SumV(V)"] -> w45
    tunnel: ["总电流(A)" "SumCurr(A)"] -> w44
    tunnel: ["外总压(V)" "SumV_Out(V)"] -> w43
    tunnel: ["平均电流(A)" "Aver_Curr(A)"] -> w42
    tunnel: ["协议版本号" "Protocol_Ver"] -> w41
    tunnel: ["波特率" "Baudrate"] -> w40
    tunnel: ["应用类型" "Application_Type"] -> w39
    tunnel: ["协议是否公开" "Protocol_Open"] -> w38
    tunnel: ["电池运行状态" "Bat_running state"] -> w37
    tunnel: ["电池充满标志位" "Bat_full_flag"] -> w36
    tunnel: ["最高电压" "Max_V"] -> w35
    tunnel: ["位置" w1210] -> w34
    tunnel: ["最低电压" "Min_V"] -> w33
    tunnel: ["位置" w1210] -> w32
    tunnel: ["最高温度" "Max_T"] -> w31
    tunnel: ["位置" w1210] -> w30
    tunnel: ["最低温度" "Min_T"] -> w29
    tunnel: ["位置" w1210] -> w28
    tunnel: ["温差" "Diff_T"] -> w27
    tunnel: ["压差" "Diff_V"] -> w26
    tunnel: ["最高内阻" "Max_R"] -> w25
    tunnel: ["位置" w1210] -> w24
    tunnel: ["最低内阻" "Min_R"] -> w23
    tunnel: ["位置" w1210] -> w22
    tunnel: ["故障信息" "Fault_Info"] -> w21
    tunnel: ["最大充电总电压" "Max_Chg_SumV"] -> w20
    tunnel: ["最大充电电流" "Max_Chg_Curr"] -> w19
    tunnel: ["充电总安时" "Total_In_Ah"] -> w18
    tunnel: ["从板监控" "Slave_Monitor"] -> w17
    tunnel: ["硬件故障" "HD_Fault"] -> w16
    tunnel: ["单体电压温度" "Cellv/Temp"] -> w15
    tunnel: ["刷新" "Refresh"] -> w14
    tunnel: ["从板板号" "Slave_No."] -> w13
    tunnel: ["硬件故障" "HD_Fault"] -> w12
    tunnel: ["单板信息" "Single board information"] -> w10
    tunnel: ["第" ""] -> w8
    tunnel: ["串" ""] -> w7
    tunnel: ["电压基准" "V_reference"] -> w5
    tunnel: ["偏差" "Offset"] -> w2
    tunnel: ["温度基准" "T_reference"] -> w4
    tunnel: ["判定" "Judge"] -> w3
    frame "中文", Default {
    }
    frame "English" {
      w1210 = "NO."
    }
  }
  n731 = control-ref of="本VI"() -> (w11:refnum<vi>)
  n732 = for {
    N: 5 -> [_]
    tunnel: w8 -> [w1247]
    tunnel: w7 -> [w1246]
    i -> [w1245]
    w1248 = 12
    n733 = for {
      N: w1248 -> [_]
      tunnel: [w1264] -> w1242 mode=indexing
      tunnel: w1245 -> [w1261]
      tunnel: w1248 -> [w1260]
      tunnel: w1246 -> [w1257]
      tunnel: w1247 -> [w1256]
      i -> [w1263]
      n734 = Multiply(x=w1261, y=w1260) -> (x*y=w1262:i32)
      n735 = Compound Arithmetic op=ADD(w1263, w1262, 1 ("值")) -> (w1258:i32)
      n736 = Number To Decimal String(number=w1258) -> (decimal integer string=w1265:string)  [unwired: 1 in]
      n737 = Concatenate Strings(w1257, w1265, w1256) -> (w1264:string)
    }
    n738 = case shown="4" w1245 {
      tunnel: [w1251 w1252 w1253 w1254 w1255] -> w1244
      frame 0, Default {
        n739 = control-ref of="1 102"() -> (w1251:refnum<vi>)
      }
      frame 1 {
        n740 = control-ref of="1 3"() -> (w1252:refnum<vi>)
      }
      frame 2 {
        n741 = control-ref of="1 4"() -> (w1253:refnum<vi>)
      }
      frame 3 {
        n742 = control-ref of="1 6"() -> (w1254:refnum<vi>)
      }
      frame 4 {
        n743 = control-ref of="1 7"() -> (w1255:refnum<vi>)
      }
    }
    n744 = property class="Clust (严格)"(reference=w1244) -> ("Controls[]"=w1243:refnum<vi>[])  [unwired: 1 in, 2 out]
    n745 = for {
      tunnel: w1243 -> [w1250] mode=indexing
      tunnel: w1242 -> [w1249] mode=indexing
      n746 = property class="Ctl"(reference=w1250, "Caption.Text"=w1249) -> ()  [unwired: 1 in, 2 out]
    }
  }
  n747 = for {
    N: 5 -> [_]
    tunnel: w8 -> [w1271]
    tunnel: w7 -> [w1270]
    i -> [w1269]
    w1272 = 12
    n748 = for {
      N: w1272 -> [_]
      tunnel: [w1288] -> w1266 mode=indexing
      tunnel: w1269 -> [w1285]
      tunnel: w1272 -> [w1284]
      tunnel: w1270 -> [w1281]
      tunnel: w1271 -> [w1280]
      i -> [w1287]
      n749 = Multiply(x=w1285, y=w1284) -> (x*y=w1286:i32)
      n750 = Compound Arithmetic op=ADD(w1287, w1286, 1 ("值")) -> (w1282:i32)
      n751 = Number To Decimal String(number=w1282) -> (decimal integer string=w1289:string)  [unwired: 1 in]
      n752 = Concatenate Strings(w1281, w1289, w1280) -> (w1288:string)
    }
    n753 = case shown="4" w1269 {
      tunnel: [w1275 w1276 w1277 w1278 w1279] -> w1268
      frame 0, Default {
        n754 = control-ref of="1"() -> (w1275:refnum<vi>)
      }
      frame 1 {
        n755 = control-ref of="2"() -> (w1276:refnum<vi>)
      }
      frame 2 {
        n756 = control-ref of="3"() -> (w1277:refnum<vi>)
      }
      frame 3 {
        n757 = control-ref of="4"() -> (w1278:refnum<vi>)
      }
      frame 4 {
        n758 = control-ref of="5"() -> (w1279:refnum<vi>)
      }
    }
    n759 = property class="Clust (严格)"(reference=w1268) -> ("Controls[]"=w1267:refnum<vi>[])  [unwired: 1 in, 2 out]
    n760 = for {
      tunnel: w1267 -> [w1274] mode=indexing
      tunnel: w1266 -> [w1273] mode=indexing
      n761 = property class="Ctl"(reference=w1274, "Caption.Text"=w1273) -> ()  [unwired: 1 in, 2 out]
    }
  }
  n762 = property on="总电压(V)" class="DigNum (严格)"("Caption.Text"=w45) -> ()  [unwired: 2 in, 2 out]
  n763 = property on="总电流(A)" class="DigNum (严格)"("Caption.Text"=w44) -> ()  [unwired: 2 in, 2 out]
  n764 = property on="外总压(V)" class="DigNum (严格)"("Caption.Text"=w43) -> ()  [unwired: 2 in, 2 out]
  n765 = property on="平均电流(A)" class="DigNum (严格)"("Caption.Text"=w42) -> ()  [unwired: 2 in, 2 out]
  n766 = property on="协议版本号" class="Str"("Caption.Text"=w41) -> ()  [unwired: 2 in, 2 out]
  n767 = property on="波特率" class="Str"("Caption.Text"=w40) -> ()  [unwired: 2 in, 2 out]
  n768 = property on="应用类型" class="Str"("Caption.Text"=w39) -> ()  [unwired: 2 in, 2 out]
  n769 = property on="协议是否公开" class="Str"("Caption.Text"=w38) -> ()  [unwired: 2 in, 2 out]
  n770 = property on="电池运行状态" class="Str"("Caption.Text"=w37) -> ()  [unwired: 2 in, 2 out]
  n771 = property on="电池充满标志位" class="Str"("Caption.Text"=w36) -> ()  [unwired: 2 in, 2 out]
  n772 = property on="最高电压" class="DigNum (严格)"("Caption.Text"=w35) -> ()  [unwired: 2 in, 2 out]
  n773 = property on="位置1" class="DigNum (严格)"("Caption.Text"=w34) -> ()  [unwired: 2 in, 2 out]
  n774 = property on="最低电压" class="DigNum (严格)"("Caption.Text"=w33) -> ()  [unwired: 2 in, 2 out]
  n775 = property on="位置2" class="DigNum (严格)"("Caption.Text"=w32) -> ()  [unwired: 2 in, 2 out]
  n776 = property on="最高温度" class="DigNum (严格)"("Caption.Text"=w31) -> ()  [unwired: 2 in, 2 out]
  n777 = property on="位置3" class="DigNum (严格)"("Caption.Text"=w30) -> ()  [unwired: 2 in, 2 out]
  n778 = property on="最低温度" class="DigNum (严格)"("Caption.Text"=w29) -> ()  [unwired: 2 in, 2 out]
  n779 = property on="位置4" class="DigNum (严格)"("Caption.Text"=w28) -> ()  [unwired: 2 in, 2 out]
  n780 = property on="压差" class="DigNum (严格)"("Caption.Text"=w26) -> ()  [unwired: 2 in, 2 out]
  n781 = property on="温差" class="DigNum (严格)"("Caption.Text"=w27) -> ()  [unwired: 2 in, 2 out]
  n782 = property on="最高内阻" class="DigNum (严格)"("Caption.Text"=w25) -> ()  [unwired: 2 in, 2 out]
  n783 = property on="位置5" class="DigNum (严格)"("Caption.Text"=w24) -> ()  [unwired: 2 in, 2 out]
  n784 = property on="最低内阻" class="DigNum (严格)"("Caption.Text"=w23) -> ()  [unwired: 2 in, 2 out]
  n785 = property on="位置6" class="DigNum (严格)"("Caption.Text"=w22) -> ()  [unwired: 2 in, 2 out]
  n786 = property on="故障信息" class="Str"("Caption.Text"=w21) -> ()  [unwired: 2 in, 2 out]
  n787 = property on="最大充电总电压" class="DigNum (严格)"("Caption.Text"=w20) -> ()  [unwired: 2 in, 2 out]
  n788 = property on="最大充电电流" class="DigNum (严格)"("Caption.Text"=w19) -> ()  [unwired: 2 in, 2 out]
  n789 = property on="充电总安时" class="DigNum (严格)"("Caption.Text"=w18) -> ()  [unwired: 2 in, 2 out]
  n790 = property on="单选选项2" class="Bool (严格)"("BoolText.Text"=w16) -> ()  [unwired: 2 in, 2 out]
  n791 = property on="单选选项1" class="Bool (严格)"("BoolText.Text"=w17) -> ()  [unwired: 2 in, 2 out]
  n792 = property on="单选选项2 2" class="Bool (严格)"("BoolText.Text"=w15) -> ()  [unwired: 2 in, 2 out]
  n793 = property on="刷新" class="Bool (严格)"("BoolText.Text"=w14) -> ()  [unwired: 2 in, 2 out]
  n794 = property on="电压基准" class="DigNum (严格)"("Caption.Text"=w5) -> ()  [unwired: 2 in, 2 out]
  n795 = property on="布尔" class="Bool (严格)"("Caption.Text"=w3) -> ()  [unwired: 2 in, 2 out]
  n796 = property on="布尔 2" class="Bool (严格)"("Caption.Text"=w3) -> ()  [unwired: 2 in, 2 out]
  n797 = property class="VI"(reference=w11, "Front Panel.Title"=w10) -> ()  [unwired: 1 in, 2 out]
  n798 = property on="偏差" class="DigNum (严格)"("Caption.Text"=w2) -> ()  [unwired: 2 in, 2 out]
  n799 = property on="偏差" class="DigNum (严格)"("Caption.Text"=w2) -> ()  [unwired: 2 in, 2 out]
  n800 = property on="从板板号 2" class="DigNum (严格)"("Caption.Text"=w13) -> ()  [unwired: 2 in, 2 out]
  n801 = property on="温度基准" class="DigNum (严格)"("Caption.Text"=w4) -> ()  [unwired: 2 in, 2 out]
  n802 = property on="硬件故障" class="Arr (严格)"("Caption.Text"=w12) -> ()  [unwired: 2 in, 2 out]
  n803 = local write "布尔 3"(TRUE ("布尔 3")) -> ()
  "单选选项2" <- FALSE ("单选选项2")
